vi "tui_DataLog Tag Manager.vi"() -> ()   [LabVIEW 2012]
doc: "Manages tags contained in the logging databases present on the connected server. This manager requires that the \"Databases Module\" is initialised on the server. The operations allowed on the selected database depend on the mode of that database. \n\nIf you find yourself repeatedly performing the same kinds of operations, e.g. because the number of tags in a database is very large, some automation might be handy. For this reason, the management operations can also be performed programatically by calling export functions of the \"Databases Module\" from a script."
uses:
  typedefs/t_Datalog Datebase Modes.ctl
  served/DataLog Database Infos_srv.ctl
  served/DataLog Tag Subset Last_srv.ctl
  served/DataLog Databases_srv.ctl
  served/DataLog Set Tag Value_srv.ctl
  served/DataLog Dump Tag Buffer_srv.ctl
  typedefs/t_DataLog Tag Manager States.ctl
  typedefs/et_DataLog Meta Tag Specifier.ctl
  library/typedefs/t_Library Session Methods.ctl
  typedefs/t_DataLog Tag Info List Methods.ctl
  clientsrv/typedefs/t_ClientSrv Access Levels.ctl
  typedefs/t_DataLog Value Types.ctl
  typedefs/t_DataLog Temporal Types.ctl
panel:
  out "dump tag buffer":T1
  in  "stats":bool
  out "set tag value":T2
  out "mode":T3
  in  "database":i32(ring)
  out "databases":T4
  out "tag subset last":T5
  out "database infos":T6
  in  "set":bool
  in  "chart":bool
  out "total tags":i32
  out "shown tags":i32
  in  "filter/subset":string(combo)
  in  "hide meta?":bool
  in  "selected":string
  in  "configure":bool
  in  "delete":bool
  in  "rename":bool
  in  "clone":bool
  in  "create meta":bool
  in  "create":bool
  in  "tag list":i32(listbox)
  in  "exit":bool
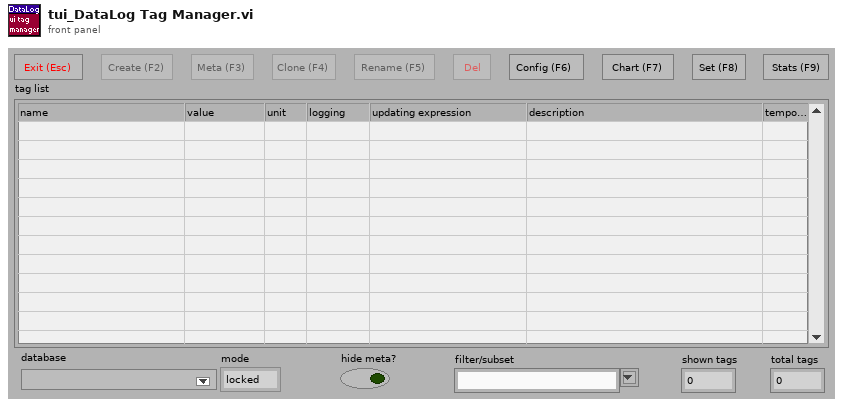
[diagram p1: front panel]
types:
  T1 = typedef "DataLog Dump Tag Buffer_srv.ctl" = refnum<vi>
  T2 = typedef "DataLog Set Tag Value_srv.ctl" = refnum<vi>
  T3 = typedef "t_Datalog Datebase Modes.ctl" = enum16{"locked", "unlocked", "live", "mirrored"}
  T4 = typedef "DataLog Databases_srv.ctl" = refnum<vi>
  T5 = typedef "DataLog Tag Subset Last_srv.ctl" = refnum<vi>
  T6 = typedef "DataLog Database Infos_srv.ctl" = refnum<vi>
  T7 = typedef "et_DataLog Meta Tag Specifier.ctl" = enum32{"warn_lo", "warn_hi", "A_lo", "A_hi", "B_lo", "B_hi", "C_lo", "C_hi", "D_lo", "D_hi", "E_lo", "E_hi", "F_lo", "F_hi", "G_lo", "G_hi", "H_lo", "H_hi", "I_lo", "I_hi", "J_lo", "J_hi", "K_lo", "K_hi", "L_lo", "L_hi", "M_lo", "M_hi", "N_lo", "N_hi", "min", "max", "not a meta"}
  T8 = typedef "t_DataLog Tag Manager States.ctl" = enum16{"empty queue", "poll list", "poll live", "resize", "set database", "get subsets", "winnow list", "filter list", "subset list", "show list", "create tag", "create meta tag", "clone tag", "rename tag", "configure tag", "chart tag", "set tag", "stat tag", "delete tag", "ablement", "initialize", "init refs", "init databases", "init persist", "cleanup", "stop"}
  T9 = typedef "t_Library Session Methods.ctl" = enum16{"run", "get arg", "set arg", "delist", "cleanup?", "start session", "stop session", "list empty?"}
  T10 = typedef "t_DataLog Tag Info List Methods.ctl" = enum16{"initialize", "create", "create empty", "rename", "delete", "test tag", "get", "get by name", "get default", "get list", "get path", "get subsets", "set subsets", "set config", "set capacity", "#tags", "go live", "set unlocked", "set mirrored"}
  T11 = typedef "t_ClientSrv Access Levels.ctl" = enum16{"observer", "operator", "local"}
  T12 = typedef "t_DataLog Temporal Types.ctl" = enum16{"set&hold", "sample", "event"}
  T13 = typedef "t_DataLog Value Types.ctl" = enum16{"number", "string"}
  T14 = typedef "eventvkey.ctl" = enum16{"ASCII", "Enter", "Return", "Shift", "Ctrl", "Alt", "Cmd", "Opt", "Caps", "NumLock", "Clear", "Break", "Up", "Down", "Left", "Right", "Insert", "Delete", "Home", "End", "PageUp", "PageDown", "Escape", "Help", "Pause", "ScrollLock", "F1", "F2", "F3", "F4", "F5", "F6", "F7", "F8", "F9", "F10", "F11", "F12", "F13", "F14", "F15", "F16", "F17", "F18", "F19", "F20", "F21", "F22", "F23", "F24", "Play", "VolumeUp", "VolumeDown", "Mute", "Two Byte Char"}
  T15 = typedef "t_DataLog Tag Config.ctl" = cluster{"name":string, "unit":string, "temporal":T12, "value":T13, "index":i32, "capacity":i32, "is meta?":bool, "mincapacity":i32, "deadband":dbl, "limit delay":dbl, "format":T16, "precision":u8, "undefine":bool, "update":bool, "update period":u16, "expression":string, "description":string, "logging algorithm":T17, "logging parameters":dbl[]}
  T16 = typedef "t_DataLog Numerical Format.ctl" = enum8{"fractional", "exponential", "engineering"}
  T17 = typedef "t_DataLog Logging Algorithms.ctl" = enum16{"nothing", "changes", "everything", "every Nth", "time threshold", "value threshold + prior", "t or v threshold", "t or v threshold + prior"}
  T18 = typedef "LVRowAndColumnUnsignedTypeDef.ctl" = cluster{"Row":u32, "Column":u32}
  T19 = typedef "t_DataLog Tag Subset.ctl" = cluster{"name":string, "tags":string[]}
  T20 = typedef "t_DataLog Point.ctl" = cluster{"time":dbl, "value":dbl}
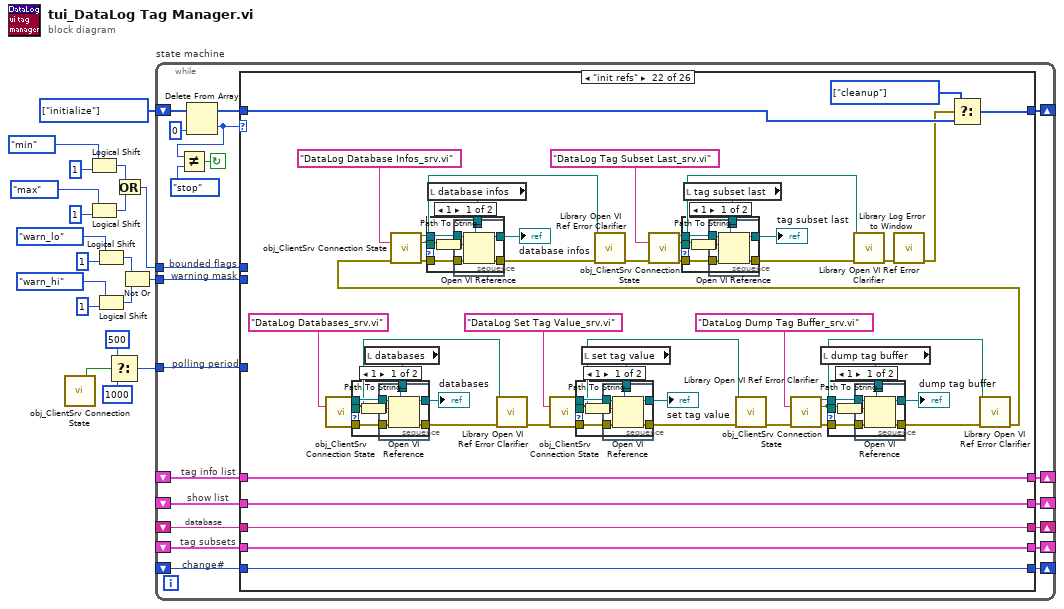
[diagram p0: block diagram]
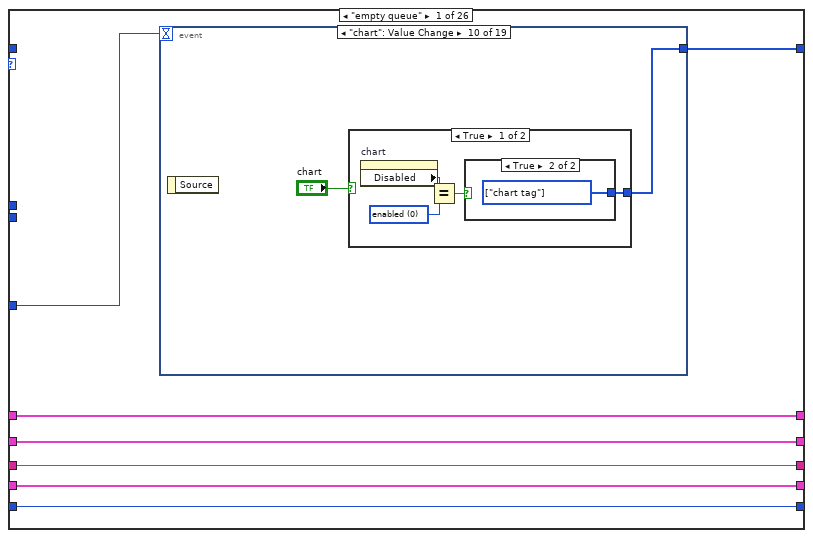
[diagram p2: hidden frame]
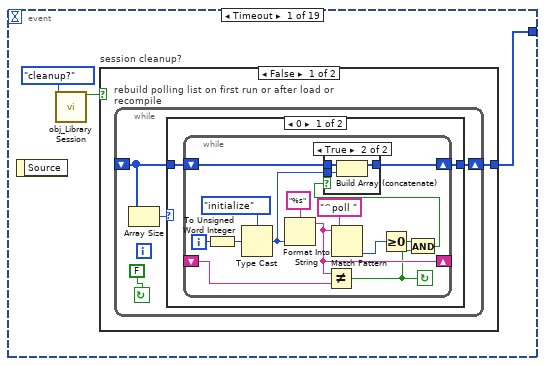
[diagram p3: hidden frame]
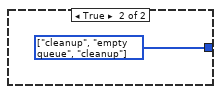
[diagram p6: hidden frame]
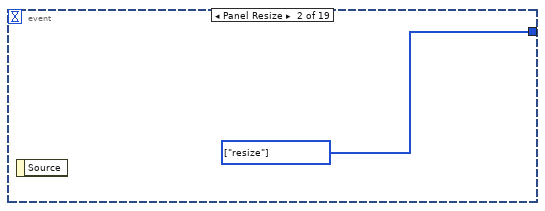
[diagram p7: hidden frame]
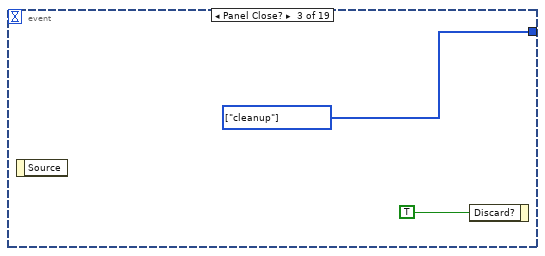
[diagram p8: hidden frame]
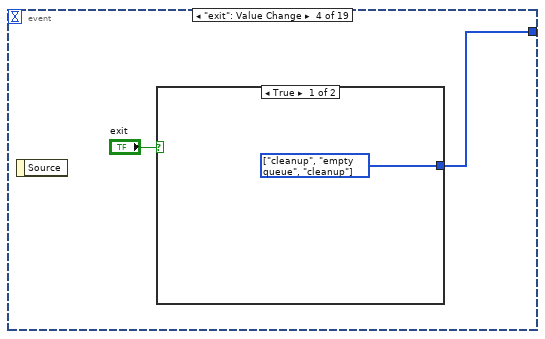
[diagram p9: hidden frame]
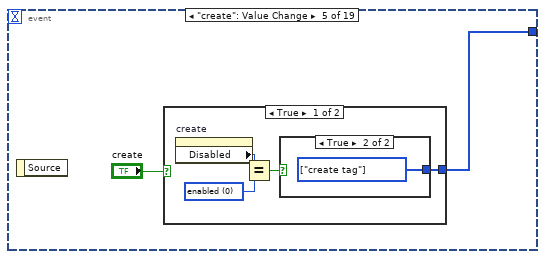
[diagram p11: hidden frame]
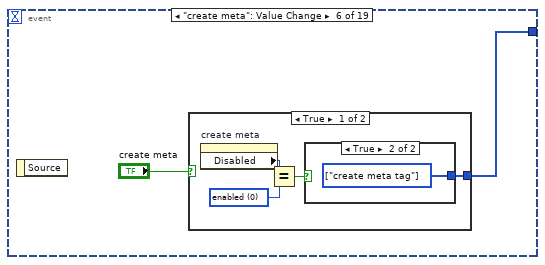
[diagram p14: hidden frame]
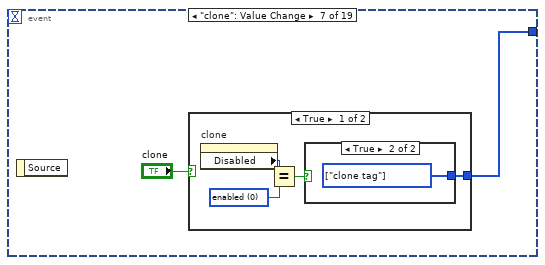
[diagram p17: hidden frame]
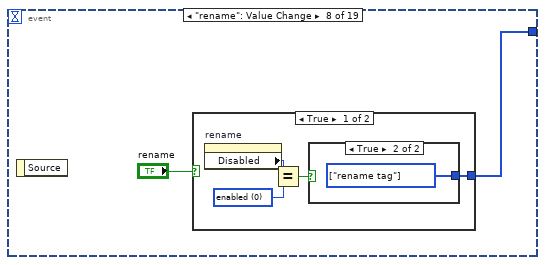
[diagram p20: hidden frame]
diagram:
  w19 = T8[] [enum."initialize"] items=["empty queue", "poll list", "poll live", "resize", "set database", "get subsets", "winnow list", "filter list", "subset list", "show list", "create tag", "create meta tag", "clone tag", "rename tag", "configure tag", "chart tag", "set tag", "stat tag", "delete tag", "ablement", "initialize", "init refs", "init databases", "init persist", "cleanup", "stop"] ("Array Constant")
  n1 = call "obj_ClientSrv Connection State.vi"() -> ("local?"=w9:bool)  [unwired: 8 in, 7 out]
  n2 = Logical Shift(y=et_DataLog_Meta_Tag_Specifier."min" ("meta specifier"), x=u32 1) -> (x << y=w6:u32)
  n3 = Logical Shift(y=et_DataLog_Meta_Tag_Specifier."max" ("meta specifier"), x=u32 1) -> (x << y=w7:u32)
  n4 = Logical Shift(y=et_DataLog_Meta_Tag_Specifier."warn_lo" ("meta specifier"), x=u32 1) -> (x << y=w14:u32)
  n5 = Logical Shift(y=et_DataLog_Meta_Tag_Specifier."warn_hi" ("meta specifier"), x=u32 1) -> (x << y=w13:u32)
  n6 = Select(t=500, s=w9, f=1000) -> (s? t:f=w8:i32)
  n7 = Or(x=w6, y=w7) -> (x .or. y?=w1:u32)
  n8 = Not Or(1:w13, 2:w14) -> (0:w12:u32)
  n9 = while "state machine" {
    shift-left: w19 -> [w36]
    shift-right: [w39] -> _
    shift-right: [w32] -> _
    shift-left: _ -> [w33]
    shift-right: [w30] -> _
    shift-left: _ -> [w31]
    tunnel: w12 -> [w29]
    tunnel: w8 -> [w27]
    shift-right: [w25] -> _
    shift-left: _ -> [w26]
    tunnel: w1 -> [w24]
    shift-right: [w23] -> _
    shift-left: _ -> [w22]
    shift-right: [w20] -> _
    shift-left: _ -> [w21]
    stop <- w38 continue-if-true
    # "change#"
    # "tag subsets"
    # "bounded flags"
    # "database"
    # "polling period"
    # "warning mask"
    # "show list"
    # "tag info list"
    n10 = Delete From Array(array=w36, index=0) -> (deleted portion=w28:T8, array with subset deleted=w35:T8[])  [unwired: 1 in]
    n11 = Not Equal?(x=w28, y=t_DataLog_Tag_Manager_States."stop" ("states")) -> (x != y?=w38:bool)
    n12 = case "Case" shown="\"init refs\"" w28 {
      tunnel: [w46 w178 w231 w303 w310 w335 w375 w391 w426 w474 w535 w599 w642 w672 w694 w734 w747 w774 w795 w844 w859 w937 w1052 w1062 w1092 w1098] -> w39
      tunnel: w35 -> [_ w179 w231 w303 w310 w334 w374 w390 w425 w473 w534 w598 w641 w671 _ w734 w745 w774 w794 w844 _ w935 w1043 w1063 _ w1098]
      tunnel: w33 -> [w45 w180 w229 w305 w315 w347 w371 _ _ w470 w539 w601 w638 w674 w697 w737 w750 w778 w797 w840 w863 w934 w1060 w1069 w1083 w1097]
      tunnel: [w45 w180 w228 w305 w315 w347 w371 w383 w421 w470 w539 w601 w638 w674 w697 w737 w750 w778 w797 w840 w863 w934 w1060 w1069 w1082 w1097] -> w32
      tunnel: w31 -> [w44 w182 w232 w304 w314 w346 w370 w385 w422 w471 w533 w595 w640 w664 w695 w735 w748 w776 w787 w842 w862 w933 w1059 w1068 w1091 w1096]
      tunnel: [w44 w181 w232 w304 w314 w346 w370 w386 w423 w471 w533 w595 w640 w664 w695 w735 w748 w776 w787 w842 w862 w933 w1059 w1068 w1086 w1096] -> w30
      tunnel: w29 -> [_ _ w227 _ _ _ _ _ _ _ _ _ _ _ _ _ _ _ _ _ _ _ _ _ _ _]
      tunnel: w27 -> [w43 _ _ _ _ _ _ _ _ _ _ _ _ _ _ _ _ _ _ _ _ _ _ _ _ _]
      tunnel: w26 -> [w42 w168 w226 w301 _ w328 w373 w379 w420 w469 w532 w594 w635 w663 w692 w727 w744 w775 w786 w818 w861 w926 w1046 w1067 w1080 w1095]
      tunnel: [w42 w168 w226 w301 w306 w328 w373 w379 w420 w469 w532 w594 w635 w663 w692 w727 w744 w775 w786 w818 w861 w926 w1046 w1067 w1080 w1095] -> w25
      tunnel: w24 -> [_ _ w225 _ _ _ _ _ _ _ _ _ _ _ _ _ _ _ _ _ _ _ _ _ _ _]
      tunnel: [w41 w167 w224 w300 w312 w339 w372 w378 w416 w468 w531 w592 w634 w662 w691 w726 w739 w764 w784 w812 w860 w920 w1047 w1066 w1071 w1094] -> w23
      tunnel: w22 -> [w41 w167 w224 w300 w312 _ w372 w378 w416 w468 w531 w592 w634 w662 w691 w726 w739 w764 w784 w812 w860 w920 w1047 w1066 w1071 w1094]
      tunnel: w21 -> [w40 w166 w223 w299 _ w329 w363 w376 w412 w467 w530 w591 w633 w661 w690 w725 w738 w763 w783 w811 w858 w919 w1045 w1064 w1070 w1093]
      tunnel: [w40 w165 w223 w299 0 ("#tags") w329 w363 w376 w412 w467 w530 w591 w633 w661 w690 w725 w738 w763 w783 w811 w858 w919 w1045 w1064 w1070 w1093] -> w20
      frame "empty queue" {
        n13 = event shown="[9] \"chart\": Value Change" {
          selector: _ -> [_ _ _ _ _ _ _ _ _ _ _ _ _ _ _ _ _ _ _]
          dyn-events: _ -> [_ _ _ _ _ _ _ _ _ _ _ _ _ _ _ _ _ _ _]
          timeout: w43 -> [_ _ _ _ _ _ _ _ _ _ _ _ _ _ _ _ _ _ _]
          tunnel: [w49 w77 w79 w81 w83 w90 w97 w104 w111 w119 w126 w133 w139 w146 w147 w148 w149 _ _] -> w46
          event Timeout {
            n14 = event-data() -> ()  [unwired: 1 in, 1 out]
            n15 = call "obj_Library Session.vi"("method"=t_Library_Session_Methods."cleanup?") -> ("cleanup/empty?"=w47:bool)  [unwired: 11 in, 3 out]
            n16 = case "session cleanup?" shown="False" w47 {
              tunnel: [w50 w76] -> w49
              frame False {
                n17 = while "rebuild polling list on first run or after load or recompile" {
                  shift-left: _ -> [w53]
                  shift-right: [w52] -> w50
                  stop <- FALSE continue-if-true
                  n18 = Array Size(array=w53) -> (size(s)=w54:i32)
                  n19 = case shown="0" w54 {
                    tunnel: [w55 w75] -> w52
                    tunnel: w53 -> [w56 w75]
                    frame 0 {
                      n20 = while {
                        shift-left: w56 -> [w65]
                        shift-right: [w63] -> w55
                        shift-left: _ -> [w67]
                        shift-right: [w62] -> _
                        i -> [w70]
                        stop <- w58 continue-if-true
                        n21 = To Unsigned Word Integer(number=w70) -> (unsigned 16bit integer=w68:u16)
                        n22 = Type Cast(type=t_DataLog_Tag_Manager_States."initialize" ("states"), x=w68) -> (*(type *) &x=w64:T8)
                        n23 = Format Into String(format string="%s" ("Format String"), w64) -> (resulting string=w62:string)  [unwired: 2 in, 1 out]
                        n24 = Not Equal?(x=w62, y=w67) -> (x != y?=w58:bool)
                        n25 = Match Pattern(string=w62, regular expression="^poll ") -> (offset past match=w60:i32)  [unwired: 1 in, 3 out]
                        n26 = Greater Or Equal To 0?(x=w60) -> (x >= 0?=w59:bool)
                        n27 = And(x=w59, y=w58) -> (x .and. y?=w57:bool)
                        n28 = case shown="True" w57 {
                          tunnel: w65 -> [w71 w74]
                          tunnel: w64 -> [_ w73]
                          tunnel: [w71 w72] -> w63
                          frame False {
                          }
                          frame True {
                            n29 = Build Array (concatenate)(w74, w73) -> (w72:T8[])
                          }
                        }
                      }
                    }
                    frame Default {
                    }
                  }
                }
              }
              frame True {
                w76 = T8[] [enum."cleanup", enum."empty queue", enum."cleanup"] items=["empty queue", "poll list", "poll live", "resize", "set database", "get subsets", "winnow list", "filter list", "subset list", "show list", "create tag", "create meta tag", "clone tag", "rename tag", "configure tag", "chart tag", "set tag", "stat tag", "delete tag", "ablement", "initialize", "init refs", "init databases", "init persist", "cleanup", "stop"] ("Array Constant")
              }
            }
          }
          event Panel Resize {
            w77 = T8[] [enum."resize"] items=["empty queue", "poll list", "poll live", "resize", "set database", "get subsets", "winnow list", "filter list", "subset list", "show list", "create tag", "create meta tag", "clone tag", "rename tag", "configure tag", "chart tag", "set tag", "stat tag", "delete tag", "ablement", "initialize", "init refs", "init databases", "init persist", "cleanup", "stop"] ("Array Constant")
            n30 = event-data() -> ()  [unwired: 1 in, 1 out]
          }
          event Panel Close? {
            w79 = T8[] [enum."cleanup"] items=["empty queue", "poll list", "poll live", "resize", "set database", "get subsets", "winnow list", "filter list", "subset list", "show list", "create tag", "create meta tag", "clone tag", "rename tag", "configure tag", "chart tag", "set tag", "stat tag", "delete tag", "ablement", "initialize", "init refs", "init databases", "init persist", "cleanup", "stop"] ("Array Constant")
            n31 = event-data() -> ()  [unwired: 1 in, 1 out]
            n32 = event-data("Discard?"=TRUE) -> ()  [unwired: 1 in, 1 out]
          }
          event "exit": Value Change {
            n33 = event-data() -> ()  [unwired: 1 in, 1 out]
            n34 = case shown="True" "exit" {
              tunnel: [w82 _] -> w81
              frame True {
                w82 = T8[] [enum."cleanup", enum."empty queue", enum."cleanup"] items=["empty queue", "poll list", "poll live", "resize", "set database", "get subsets", "winnow list", "filter list", "subset list", "show list", "create tag", "create meta tag", "clone tag", "rename tag", "configure tag", "chart tag", "set tag", "stat tag", "delete tag", "ablement", "initialize", "init refs", "init databases", "init persist", "cleanup", "stop"] ("Array Constant")
              }
              frame False {
              }
            }
          }
          event "create": Value Change {
            n35 = event-data() -> ()  [unwired: 1 in, 1 out]
            n36 = case shown="True" "create" {
              tunnel: [w88 _] -> w83
              frame True {
                w87 = u8 0 items=["enabled", "disabled", "grayed"] ("disabled state")
                n37 = property on="create" class="Bool"() -> ("Disabled"=w86:u8)  [unwired: 2 in, 2 out]
                n38 = Equal?(x=w86, y=w87) -> (x = y?=w85:bool)
                n39 = case shown="True" w85 {
                  tunnel: [_ w89] -> w88
                  frame False {
                  }
                  frame True {
                    w89 = T8[] [enum."create tag"] items=["empty queue", "poll list", "poll live", "resize", "set database", "get subsets", "winnow list", "filter list", "subset list", "show list", "create tag", "create meta tag", "clone tag", "rename tag", "configure tag", "chart tag", "set tag", "stat tag", "delete tag", "ablement", "initialize", "init refs", "init databases", "init persist", "cleanup", "stop"] ("Array Constant")
                  }
                }
              }
              frame False {
              }
            }
          }
          event "create meta": Value Change {
            n40 = event-data() -> ()  [unwired: 1 in, 1 out]
            n41 = case shown="True" "create meta" {
              tunnel: [w95 _] -> w90
              frame True {
                w94 = u8 0 items=["enabled", "disabled", "grayed"] ("disabled state")
                n42 = property on="create meta" class="Bool"() -> ("Disabled"=w93:u8)  [unwired: 2 in, 2 out]
                n43 = Equal?(x=w93, y=w94) -> (x = y?=w92:bool)
                n44 = case shown="True" w92 {
                  tunnel: [_ w96] -> w95
                  frame False {
                  }
                  frame True {
                    w96 = T8[] [enum."create meta tag"] items=["empty queue", "poll list", "poll live", "resize", "set database", "get subsets", "winnow list", "filter list", "subset list", "show list", "create tag", "create meta tag", "clone tag", "rename tag", "configure tag", "chart tag", "set tag", "stat tag", "delete tag", "ablement", "initialize", "init refs", "init databases", "init persist", "cleanup", "stop"] ("Array Constant")
                  }
                }
              }
              frame False {
              }
            }
          }
          event "clone": Value Change {
            n45 = event-data() -> ()  [unwired: 1 in, 1 out]
            n46 = case shown="True" "clone" {
              tunnel: [w102 _] -> w97
              frame True {
                w101 = u8 0 items=["enabled", "disabled", "grayed"] ("disabled state")
                n47 = property on="clone" class="Bool"() -> ("Disabled"=w100:u8)  [unwired: 2 in, 2 out]
                n48 = Equal?(x=w100, y=w101) -> (x = y?=w99:bool)
                n49 = case shown="True" w99 {
                  tunnel: [_ w103] -> w102
                  frame False {
                  }
                  frame True {
                    w103 = T8[] [enum."clone tag"] items=["empty queue", "poll list", "poll live", "resize", "set database", "get subsets", "winnow list", "filter list", "subset list", "show list", "create tag", "create meta tag", "clone tag", "rename tag", "configure tag", "chart tag", "set tag", "stat tag", "delete tag", "ablement", "initialize", "init refs", "init databases", "init persist", "cleanup", "stop"] ("Array Constant")
                  }
                }
              }
              frame False {
              }
            }
          }
          event "rename": Value Change {
            n50 = event-data() -> ()  [unwired: 1 in, 1 out]
            n51 = case shown="True" "rename" {
              tunnel: [w109 _] -> w104
              frame True {
                w108 = u8 0 items=["enabled", "disabled", "grayed"] ("disabled state")
                n52 = property on="rename" class="Bool"() -> ("Disabled"=w107:u8)  [unwired: 2 in, 2 out]
                n53 = Equal?(x=w107, y=w108) -> (x = y?=w106:bool)
                n54 = case shown="True" w106 {
                  tunnel: [_ w110] -> w109
                  frame False {
                  }
                  frame True {
                    w110 = T8[] [enum."rename tag"] items=["empty queue", "poll list", "poll live", "resize", "set database", "get subsets", "winnow list", "filter list", "subset list", "show list", "create tag", "create meta tag", "clone tag", "rename tag", "configure tag", "chart tag", "set tag", "stat tag", "delete tag", "ablement", "initialize", "init refs", "init databases", "init persist", "cleanup", "stop"] ("Array Constant")
                  }
                }
              }
              frame False {
              }
            }
          }
          event "configure": Value Change {
            n55 = event-data() -> ()  [unwired: 1 in, 1 out]
            n56 = case shown="True" "configure" {
              tunnel: [w116 _] -> w111
              frame True {
                w115 = u8 0 items=["enabled", "disabled", "grayed"] ("disabled state")
                n57 = property on="configure" class="Bool"() -> ("Disabled"=w114:u8)  [unwired: 2 in, 2 out]
                n58 = Equal?(x=w114, y=w115) -> (x = y?=w113:bool)
                n59 = case shown="True" w113 {
                  tunnel: [_ w117] -> w116
                  frame False {
                  }
                  frame True {
                    w117 = T8[] [enum."configure tag"] items=["empty queue", "poll list", "poll live", "resize", "set database", "get subsets", "winnow list", "filter list", "subset list", "show list", "create tag", "create meta tag", "clone tag", "rename tag", "configure tag", "chart tag", "set tag", "stat tag", "delete tag", "ablement", "initialize", "init refs", "init databases", "init persist", "cleanup", "stop"] ("Array Constant")
                  }
                }
              }
              frame False {
              }
            }
          }
          event "chart": Value Change {
            n60 = event-data() -> ()  [unwired: 1 in, 1 out]
            n61 = case shown="True" "chart" {
              tunnel: [w123 _] -> w119
              frame True {
                w122 = u8 0 items=["enabled", "disabled", "grayed"] ("disabled state")
                n62 = property on="chart" class="Bool"() -> ("Disabled"=w121:u8)  [unwired: 2 in, 2 out]
                n63 = Equal?(x=w121, y=w122) -> (x = y?=w120:bool)
                n64 = case shown="True" w120 {
                  tunnel: [_ w124] -> w123
                  frame False {
                  }
                  frame True {
                    w124 = T8[] [enum."chart tag"] items=["empty queue", "poll list", "poll live", "resize", "set database", "get subsets", "winnow list", "filter list", "subset list", "show list", "create tag", "create meta tag", "clone tag", "rename tag", "configure tag", "chart tag", "set tag", "stat tag", "delete tag", "ablement", "initialize", "init refs", "init databases", "init persist", "cleanup", "stop"] ("Array Constant")
                  }
                }
              }
              frame False {
              }
            }
          }
          event "set": Value Change {
            n65 = event-data() -> ()  [unwired: 1 in, 1 out]
            n66 = case shown="True" "set" {
              tunnel: [w130 _] -> w126
              frame True {
                w129 = u8 0 items=["enabled", "disabled", "grayed"] ("disabled state")
                n67 = property on="set" class="Bool"() -> ("Disabled"=w128:u8)  [unwired: 2 in, 2 out]
                n68 = Equal?(x=w128, y=w129) -> (x = y?=w127:bool)
                n69 = case shown="True" w127 {
                  tunnel: [_ w131] -> w130
                  frame False {
                  }
                  frame True {
                    w131 = T8[] [enum."set tag"] items=["empty queue", "poll list", "poll live", "resize", "set database", "get subsets", "winnow list", "filter list", "subset list", "show list", "create tag", "create meta tag", "clone tag", "rename tag", "configure tag", "chart tag", "set tag", "stat tag", "delete tag", "ablement", "initialize", "init refs", "init databases", "init persist", "cleanup", "stop"] ("Array Constant")
                  }
                }
              }
              frame False {
              }
            }
          }
          event "stats": Value Change {
            n70 = event-data() -> ()  [unwired: 1 in, 1 out]
            n71 = case shown="True" "stats" {
              tunnel: [w137 _] -> w133
              frame True {
                w136 = u8 0 items=["enabled", "disabled", "grayed"] ("disabled state")
                n72 = property on="stats" class="Bool"() -> ("Disabled"=w135:u8)  [unwired: 2 in, 2 out]
                n73 = Equal?(x=w135, y=w136) -> (x = y?=w134:bool)
                n74 = case shown="True" w134 {
                  tunnel: [_ w138] -> w137
                  frame False {
                  }
                  frame True {
                    w138 = T8[] [enum."stat tag"] items=["empty queue", "poll list", "poll live", "resize", "set database", "get subsets", "winnow list", "filter list", "subset list", "show list", "create tag", "create meta tag", "clone tag", "rename tag", "configure tag", "chart tag", "set tag", "stat tag", "delete tag", "ablement", "initialize", "init refs", "init databases", "init persist", "cleanup", "stop"] ("Array Constant")
                  }
                }
              }
              frame False {
              }
            }
          }
          event "delete": Value Change {
            n75 = event-data() -> ()  [unwired: 1 in, 1 out]
            n76 = case shown="True" "delete" {
              tunnel: [w144 _] -> w139
              frame True {
                w143 = u8 0 items=["enabled", "disabled", "grayed"] ("disabled state")
                n77 = property on="delete" class="Bool"() -> ("Disabled"=w142:u8)  [unwired: 2 in, 2 out]
                n78 = Equal?(x=w142, y=w143) -> (x = y?=w141:bool)
                n79 = case shown="True" w141 {
                  tunnel: [_ w145] -> w144
                  frame False {
                  }
                  frame True {
                    w145 = T8[] [enum."delete tag"] items=["empty queue", "poll list", "poll live", "resize", "set database", "get subsets", "winnow list", "filter list", "subset list", "show list", "create tag", "create meta tag", "clone tag", "rename tag", "configure tag", "chart tag", "set tag", "stat tag", "delete tag", "ablement", "initialize", "init refs", "init databases", "init persist", "cleanup", "stop"] ("Array Constant")
                  }
                }
              }
              frame False {
              }
            }
          }
          event "tag list": Value Change {
            w146 = T8[] [enum."ablement"] items=["empty queue", "poll list", "poll live", "resize", "set database", "get subsets", "winnow list", "filter list", "subset list", "show list", "create tag", "create meta tag", "clone tag", "rename tag", "configure tag", "chart tag", "set tag", "stat tag", "delete tag", "ablement", "initialize", "init refs", "init databases", "init persist", "cleanup", "stop"] ("Array Constant")
            n80 = event-data() -> ()  [unwired: 1 in, 1 out]
          }
          event "hide meta?": Value Change {
            w147 = T8[] [enum."winnow list"] items=["empty queue", "poll list", "poll live", "resize", "set database", "get subsets", "winnow list", "filter list", "subset list", "show list", "create tag", "create meta tag", "clone tag", "rename tag", "configure tag", "chart tag", "set tag", "stat tag", "delete tag", "ablement", "initialize", "init refs", "init databases", "init persist", "cleanup", "stop"] ("Array Constant")
            n81 = event-data() -> ()  [unwired: 1 in, 1 out]
          }
          event "filter/subset": Value Change {
            w148 = T8[] [enum."winnow list"] items=["empty queue", "poll list", "poll live", "resize", "set database", "get subsets", "winnow list", "filter list", "subset list", "show list", "create tag", "create meta tag", "clone tag", "rename tag", "configure tag", "chart tag", "set tag", "stat tag", "delete tag", "ablement", "initialize", "init refs", "init databases", "init persist", "cleanup", "stop"] ("Array Constant")
            n82 = event-data() -> ()  [unwired: 1 in, 1 out]
          }
          event "database": Value Change {
            w149 = T8[] [enum."set database", enum."get subsets", enum."poll list"] items=["empty queue", "poll list", "poll live", "resize", "set database", "get subsets", "winnow list", "filter list", "subset list", "show list", "create tag", "create meta tag", "clone tag", "rename tag", "configure tag", "chart tag", "set tag", "stat tag", "delete tag", "ablement", "initialize", "init refs", "init databases", "init persist", "cleanup", "stop"] ("Array Constant")
            n83 = event-data() -> ()  [unwired: 1 in, 1 out]
          }
          event Key Down? {
            n84 = event-data() -> ("VKey"=w150:T14, "FocusObj"=w151:refnum<vi>)  [unwired: 1 in]
            n85 = call <vilib>:"compatReturnToEnter.vi"("VKey"=w150) -> ("VKey"=w153:T14)
            n86 = case shown="\"Up\", \"Down\"" w153 {
              tunnel: [_ TRUE _] -> w152
              tunnel: w151 -> [w157 _ _]
              frame "Up", "Down" {
                n87 = Type Cast(type=u32 0, x=w157) -> (*(type *) &x=w155:u32)
                n88 = Equal To 0?(x=w155) -> (x = 0?=w154:bool)
                n89 = case shown="True" w154 {
                  frame False {
                  }
                  frame True {
                    n90 = property on="tag list" class="MCListbox (strict)"("Key Focus"=TRUE) -> ()  [unwired: 2 in, 2 out]
                  }
                }
              }
              frame "F1" {
                n91 = call "Library Show Help.vi"() -> ()  [unwired: 1 in]
              }
              frame Default {
              }
            }
            n92 = event-data("Discard?"=w152) -> ()  [unwired: 1 in, 1 out]
          }
          event event type 5.0.x8000000b {
            n93 = event-data() -> ("VKey"=w160:T14)  [unwired: 1 in]
            n94 = call <vilib>:"compatReturnToEnter.vi"("VKey"=w160) -> ("VKey"=w162:T14)
            n95 = case shown="\"F1\"" w162 {
              tunnel: [TRUE _] -> w161
              frame "F1" {
              }
              frame Default {
              }
            }
            n96 = event-data("Discard?"=w161) -> ()  [unwired: 1 in, 1 out]
          }
        }
      }
      frame "poll list" {
        n97 = local read "database infos"() -> (w172:T6)
        n98 = call "obj_ClientSrv Client Access State.vi"() -> ("certificate"=w170:string, "error out"=w173:errorcluster)  [unwired: 14 in]
        n99 = call-by-ref "?"(reference=w172, error in=w173, "method"=t_DataLog_Tag_Info_List_Methods."get list", "meta specifier (not a meta)"=w166, "certificate in"=w170, "database (current)"=w168) -> (error out=w174:errorcluster, "mode"=w176:T3, "tag config list"=w175:T15[], "#tags/change#"=w164:i32, 15:"error out"=w171:errorcluster)  [unwired: 6 in, 3 out]
        n100 = call "Library Remote Call Error Merger.vi"("call by reference node error"=w174, "called VI error (no error)"=w171) -> ("error out"=w169:errorcluster)  [unwired: 13 in]
        n101 = case shown="No Error" w169 {
          selector: w169 -> [_ w220]
          tunnel: w182 -> [w192 w221]
          tunnel: [w191 w221] -> w181
          tunnel: w179 -> [w190 _]
          tunnel: [w189 w222] -> w178
          tunnel: w176 -> [w188 _]
          tunnel: w175 -> [w187 _]
          tunnel: w166 -> [w185 w219]
          tunnel: [w184 w219] -> w165
          tunnel: w164 -> [w183 _]
          frame No Error {
            n102 = Not Equal?(x=w183, y=w185) -> (x != y?=w194:bool)
            n103 = Equal To 0?(x=w185) -> (x = 0?=w186:bool)
            n104 = Or(x=w194, y=w186) -> (x .or. y?=w193:bool)
            n105 = case shown="False" w193 {
              tunnel: [w201 w215] -> w191
              tunnel: w187 -> [_ w215]
              tunnel: w192 -> [w201 _]
              tunnel: w190 -> [w198 w217]
              tunnel: w188 -> [w200 w218]
              tunnel: [w197 w216] -> w189
              tunnel: w185 -> [w195 _]
              tunnel: [w195 w213] -> w184
              tunnel: w183 -> [_ w213]
              frame False {
                n106 = local read "mode"() -> (w196:T3)
                n107 = Not Equal?(x=w200, y=w196) -> (x != y?=w199:bool)
                n108 = case shown="True" w199 {
                  tunnel: w200 -> [_ w203]
                  tunnel: w198 -> [w202 w205]
                  tunnel: [w202 w204] -> w197
                  frame False {
                  }
                  frame True {
                    n109 = case shown="\"locked\", \"unlocked\", \"mirrored\"" w203 {
                      tunnel: w205 -> [w207 w210]
                      tunnel: [w206 w209] -> w204
                      frame "locked", "unlocked", "mirrored" {
                        n110 = Build Array (concatenate)(t_DataLog_Tag_Manager_States."show list" ("states"), w207) -> (w206:T8[])
                      }
                      frame "live" {
                        n111 = Build Array (concatenate)(t_DataLog_Tag_Manager_States."ablement" ("states"), w210) -> (w209:T8[])
                      }
                    }
                    "mode" <- w203
                  }
                }
              }
              frame True {
                w212 = T8[] [enum."get subsets", enum."winnow list"] items=["empty queue", "poll list", "poll live", "resize", "set database", "get subsets", "winnow list", "filter list", "subset list", "show list", "create tag", "create meta tag", "clone tag", "rename tag", "configure tag", "chart tag", "set tag", "stat tag", "delete tag", "ablement", "initialize", "init refs", "init databases", "init persist", "cleanup", "stop"] ("Array Constant")
                # "might be the subsets that have changed"
                n112 = local write "mode"(w218) -> ()
                n113 = Array Size(array=w215) -> (size(s)=→"total tags":i32)
                n114 = Build Array (concatenate)(w212, w217) -> (w216:T8[])
              }
            }
          }
          frame Error {
            w222 = T8[] [enum."cleanup"] items=["empty queue", "poll list", "poll live", "resize", "set database", "get subsets", "winnow list", "filter list", "subset list", "show list", "create tag", "create meta tag", "clone tag", "rename tag", "configure tag", "chart tag", "set tag", "stat tag", "delete tag", "ablement", "initialize", "init refs", "init databases", "init persist", "cleanup", "stop"] ("Array Constant")
            n115 = call "Library Log Error to Window.vi"("error in (no error)"=w220) -> ()  [unwired: 13 in, 2 out]
          }
        }
      }
      frame "poll live" {
        n116 = local read "mode"() -> (w230:T3)
        n117 = case shown="\"live\"" w230 {
          tunnel: w229 -> [w233 w237]
          tunnel: [w233 w234] -> w228
          tunnel: w227 -> [_ w236]
          tunnel: w225 -> [_ w235]
          frame Default {
          }
          frame "live" {
            n118 = stacked-sequence {
              tunnel: w237 -> [_ w248 _]
              tunnel: w236 -> [_ w257 _]
              tunnel: w235 -> [_ w242 _]
              tunnel: [_ w240 _] -> w234
              frame #0 {
                n119 = property class="VI"() -> ("Front Panel"=w238:refnum<vi>)  [unwired: 2 in, 2 out]
                n120 = property class="Pnl"(reference=w238, "Defer Panel Updates"=TRUE) -> ()  [unwired: 1 in, 2 out]
              }
              frame #1 {
                # "ignore error since\ndatabase might\nbe switching\nmodes."
                n121 = property on="tag list" class="MCListbox (strict)"() -> ("Item Names"=w262:string[][], "Top Left Visible Cell"=w258:T18, "Number of Rows"=w259:u32)  [unwired: 2 in, 2 out]
                n122 = local read "tag subset last"() -> (w255:T5)
                n123 = To Long Integer(number=w259) -> (32bit integer=w244:i32)
                n124 = Unbundle(w258) -> ("Row"=w260:u32)  [unwired: 1 out]
                n125 = Array Size(array=w248) -> (size(s)=w246:i32)
                n126 = To Long Integer(number=w260) -> (32bit integer=w247:i32)
                n127 = Subtract(x=w246, y=w247) -> (x-y=w243:i32)
                n128 = Max & Min(x=w244, y=w243) -> (min(x,y)=w245:i32)  [unwired: 1 out]
                n129 = call "obj_ClientSrv Client Access State.vi"() -> ("certificate"=w254:string, "error out"=w252:errorcluster)  [unwired: 14 in]
                n130 = for {
                  N: w245 -> [_]
                  shift-right: [w294] -> w241
                  shift-left: w248 -> [w294]
                  tunnel: [w293] -> w253 mode=indexing
                  tunnel: [w292] -> w263 mode=indexing
                  tunnel: w247 -> [w291]
                  i -> [w296]
                  n131 = Add(x=w291, y=w296) -> (x+y=w292:i32)
                  n132 = Index Array(array=w294, index=w292) -> (element=w295:T15)
                  n133 = Unbundle By Name(w295) -> ("index"=w293:i32)
                }
                n134 = call-by-ref "?"(reference=w255, error in=w252, "subset indices"=w253, "certificate"=w254) -> (error out=w251:errorcluster, "values"=w250:dbl[], "meta masks"=w249:u32[])  [unwired: 11 in, 2 out]
                n135 = call "Library Remote Call Error Merger.vi"("call by reference node error"=w251) -> ("error out"=w256:errorcluster)  [unwired: 14 in]
                n136 = call "Library Log Error to Window.vi"("error in (no error)"=w256) -> ()  [unwired: 13 in, 2 out]
                n137 = for {
                  tunnel: w263 -> [w266] mode=indexing
                  tunnel: w250 -> [w265] mode=indexing
                  shift-right: [w277] -> w261
                  shift-left: w262 -> [w274]
                  tunnel: w249 -> [w272] mode=indexing
                  tunnel: w257 -> [w271]
                  tunnel: w242 -> [w268]
                  shift-right: [w267] -> w240
                  shift-left: w241 -> [w267]
                  n138 = case shown="Default" w272 {
                    selector: w272 -> [w280 _]
                    tunnel: w271 -> [w282 _]
                    tunnel: [w281 u32 15790320] -> w270
                    tunnel: w268 -> [w279 _]
                    frame Default {
                      n139 = And(x=w280, y=w279) -> (x .and. y?=w278:u32)
                      n140 = case shown="0" w278 {
                        tunnel: w280 -> [w286 _]
                        tunnel: w282 -> [w285 _]
                        tunnel: [w283 u32 16711935] -> w281
                        frame 0 {
                          n141 = And(x=w286, y=w285) -> (x .and. y?=w284:u32)
                          n142 = case shown="0" w284 {
                            tunnel: [u32 16727100 u32 16744448] -> w283
                            frame Default {
                            }
                            frame 0 {
                            }
                          }
                        }
                        frame Default {
                        }
                      }
                    }
                    frame 0 {
                    }
                  }
                  n143 = Index Array(array=w267, index=w266) -> (element=w264:T15)
                  n144 = Bundle(w266, "x+y"=1) -> (w269:cluster{i32, "x+y":i32})  [unwired: 1 in]
                  n145 = call "DataLog Format Point Value.vi"("value"=w265, "tag config"=w264) -> ("formatted value"=w275:string)  [unwired: 13 in]
                  n146 = property on="tag list" class="MCListbox (strict)"("Active Cell:Active Cell"=w269, "Active Cell:Cell Background Color"=w270) -> ()  [unwired: 2 in, 2 out]
                  n147 = Replace Array Subset(array=w274, new element=w275, index (row)=w266, index (col)=1 ("disabled index (col)")) -> (w277:string[][])
                }
                n148 = property on="tag list" class="MCListbox (strict)"("Item Names"=w261) -> ()  [unwired: 2 in, 2 out]
              }
              frame #2 {
                n149 = property class="VI"() -> ("Front Panel"=w297:refnum<vi>)  [unwired: 2 in, 2 out]
                n150 = property class="Pnl"(reference=w297, "Defer Panel Updates"=FALSE) -> ()  [unwired: 1 in, 2 out]
              }
            }
          }
        }
      }
      frame "resize" {
        n151 = control-ref of="tag list"() -> (w302:refnum<vi>)
        n152 = call "Library MCListBox Resizer.vi"("MCListbox Refnum"=w302) -> ()  [unwired: 15 in]
      }
      frame "set database" {
        n153 = property on="database" class="Ring (strict)"() -> ("Strings []"=w308:string[])  [unwired: 2 in, 2 out]
        n154 = Index Array(array=w308, index="database") -> (element=w307:string)
        n155 = Empty String/Path?(string/path=w307) -> (empty?=w309:bool)
        n156 = case shown="True" w309 {
          tunnel: w308 -> [_ w319]
          tunnel: w307 -> [w316 _]
          tunnel: [w316 w318] -> w306
          frame False {
          }
          frame True {
            w317 = 0 ("index")
            n157 = Index Array(array=w319, index=w317) -> (element=w318:string)
            n158 = local write "database"(w317) -> ()
          }
        }
      }
      frame "get subsets" {
        w333 = T8[] [enum."cleanup"] items=["empty queue", "poll list", "poll live", "resize", "set database", "get subsets", "winnow list", "filter list", "subset list", "show list", "create tag", "create meta tag", "clone tag", "rename tag", "configure tag", "chart tag", "set tag", "stat tag", "delete tag", "ablement", "initialize", "init refs", "init databases", "init persist", "cleanup", "stop"] ("Array Constant")
        w325 = "~`&%" ("string")
        n159 = local read "database infos"() -> (w342:T6)
        n160 = call "obj_ClientSrv Client Access State.vi"() -> ("certificate"=w340:string, "error out"=w343:errorcluster)  [unwired: 14 in]
        n161 = call-by-ref "?"(reference=w342, error in=w343, "method"=t_DataLog_Tag_Info_List_Methods."get subsets", "certificate in"=w340, "database (current)"=w328) -> (error out=w344:errorcluster, "subsets out"=w339:T19[], 15:"error out"=w341:errorcluster)  [unwired: 7 in, 5 out]
        n162 = local read "filter/subset"() -> (w323:string)
        n163 = call "Library Remote Call Error Merger.vi"("call by reference node error"=w344, "called VI error (no error)"=w341) -> ("error out"=w337:errorcluster)  [unwired: 13 in]
        n164 = call "Library Log Error to Window.vi"("error in (no error)"=w337) -> ("dup error"=w336:errorcluster)  [unwired: 13 in, 1 out]
        n165 = String Subset(string=w323, length (rest)=4 ("length (rest)")) -> (substring=w326:string)  [unwired: 1 in]
        n166 = Not Equal?(x=w325, y=w326) -> (x != y?=w324:bool)
        n167 = Select(t=w323, s=w324, f="") -> (s? t:f=w322:string)
        n168 = for {
          tunnel: w339 -> [w360] mode=indexing
          shift-right: [w356] -> w331
          shift-left: cluster{"String":string, "Value":string} {"String"="all tags", "Value"=""} -> [w356]
          tunnel: [w355] -> w332 mode=indexing
          shift-right: [w350] -> w320
          shift-left: w322 -> [w348]
          tunnel: w323 -> [w349]
          tunnel: w325 -> [w352]
          n169 = Unbundle By Name(w360) -> ("name"=w357:string)
          n170 = Concatenate Strings(w352, w357) -> (w353:string)
          n171 = Equal?(x=w353, y=w349) -> (x = y?=w351:bool)
          n172 = Concatenate Strings("subset \"" ("string"), w357, "\"" ("string")) -> (w354:string)
          n173 = Bundle By Name(cluster=w356, "String"=w354, "Value"=w353) -> (w355:cluster{"String":string, "Value":string})
          n174 = Select(t=w349, s=w351, f=w348) -> (s? t:f=w350:string)
        }
        n175 = Build Array (concatenate)(w331, w332) -> (w330:cluster{"String":string, "Value":string}[])
        n176 = property on="filter/subset" class="CmbBox"("Strings And Values []"=w330, "Value"=w320) -> ()  [unwired: 2 in, 2 out]
        n177 = Select(t=w333, s=w336, f=w334) -> (s? t:f=w335:T8[])
      }
      frame "winnow list" {
        n178 = String Subset(string="filter/subset", length (rest)=4 ("length (rest)")) -> (substring=w367:string)  [unwired: 1 in]
        n179 = Equal?(x=w367, y="~`&%" ("string")) -> (x = y?=w365:bool)
        n180 = Select(t=t_DataLog_Tag_Manager_States."subset list" ("states"), s=w365, f=t_DataLog_Tag_Manager_States."filter list" ("states")) -> (s? t:f=w364:T8)
        n181 = Build Array (concatenate)(w364, w374) -> (w375:T8[])
      }
      frame "filter list" {
        n182 = local read "filter/subset"() -> (w377:string)
        n183 = Array Size(array=w385) -> (size(s)=w384:i32)
        n184 = call "Library Wildcards to Regular.vi"("wildcards"=w377) -> ("regular expression"=w380:string)  [unwired: 4 in]
        n185 = for {
          N: w384 -> [_]
          shift-right: [w398] -> w381
          shift-left: i32[] [] -> [w399]
          shift-right: [w407] -> w387
          shift-left: w385 -> [w407]
          tunnel: w380 -> [w396]
          i -> [w397]
          n186 = Index Array(array=w407, index=w397) -> (element=w406:T15)
          n187 = Unbundle By Name(w406) -> ("is meta?"=w404:bool, "name"=w405:string)
          n188 = Compound Arithmetic op=OR(invert "hide meta?", invert w404) -> (w401:bool)
          n189 = Match Pattern(string=w405, regular expression=w396) -> (offset past match=w395:i32)  [unwired: 1 in, 3 out]
          n190 = Greater Or Equal To 0?(x=w395) -> (x >= 0?=w402:bool)
          n191 = And(x=w401, y=w402) -> (x .and. y?=w400:bool)
          n192 = case shown="True" w400 {
            tunnel: w399 -> [w408 w411]
            tunnel: [w408 w410] -> w398
            tunnel: w397 -> [_ w409]
            frame False {
            }
            frame True {
              n193 = Build Array (concatenate)(w411, w409) -> (w410:i32[])
            }
          }
        }
        n194 = for {
          tunnel: w381 -> [w394] mode=indexing
          shift-right: [w393] -> w386
          shift-left: w387 -> [w393]
          tunnel: [w392] -> w383 mode=indexing
          n195 = Index Array(array=w393, index=w394) -> (element=w392:T15)
        }
        n196 = Array Size(array=w381) -> (size(s)=→"shown tags":i32)
        n197 = Build Array (concatenate)(t_DataLog_Tag_Manager_States."show list" ("states"), w390) -> (w391:T8[])
      }
      frame "subset list" {
        n198 = for {
          tunnel: w416 -> [w466] mode=indexing
          tunnel: [w465] -> w418 mode=indexing
          n199 = Unbundle By Name(w466) -> ("name"=w465:string)
        }
        n200 = local read "filter/subset"() -> (w414:string)
        n201 = String Subset(string=w414, offset (0)=4) -> (substring=w417:string)  [unwired: 1 in]
        n202 = Search 1D Array(1D array=w418, element=w417) -> (index of element=w415:i32)  [unwired: 1 in]
        n203 = Less Than 0?(x=w415) -> (x < 0?=w413:bool)
        n204 = case "selected subset no longer present?" shown="False" w413 {
          tunnel: [w439 w464] -> w423
          tunnel: w422 -> [w438 w464]
          tunnel: [w436 w464] -> w421
          tunnel: w416 -> [w433 _]
          tunnel: w415 -> [w430 _]
          frame False {
            # "avoid LV7 bug"
            n205 = Index Array(array=w433, index=w430) -> (element=w432:T19)
            n206 = Array Size(array=w438) -> (size(s)=w437:i32)
            n207 = Unbundle By Name(w432) -> ("tags"=w431:string[])
            n208 = for {
              N: w437 -> [_]
              shift-right: [w453] -> w435
              shift-left: cluster{"index of element":i32, i32}[] [] -> [w454]
              shift-right: [w458] -> w440
              shift-left: w438 -> [w458]
              tunnel: w431 -> [w450]
              i -> [w446]
              n209 = Index Array(array=w458, index=w446) -> (element=w457:T15)
              n210 = local read "hide meta?"() -> (w452:bool)
              n211 = Unbundle By Name(w457) -> ("is meta?"=w456:bool, "name"=w451:string)
              n212 = Search 1D Array(1D array=w450, element=w451) -> (index of element=w447:i32)  [unwired: 1 in]
              n213 = Compound Arithmetic op=OR(invert w452, invert w456) -> (w455:bool)
              n214 = Greater Or Equal To 0?(x=w447) -> (x >= 0?=w448:bool)
              n215 = Bundle("index of element"=w447, w446) -> (w445:cluster{"index of element":i32, i32})  [unwired: 1 in]
              n216 = And(x=w455, y=w448) -> (x .and. y?=w449:bool)
              n217 = case shown="True" w449 {
                tunnel: w454 -> [w459 w460]
                tunnel: [w459 w462] -> w453
                tunnel: w445 -> [_ w461]
                frame False {
                }
                frame True {
                  n218 = Build Array (concatenate)(w460, w461) -> (w462:cluster{"index of element":i32, i32}[])
                }
              }
            }
            n219 = Sort 1D Array(array=w435) -> (sorted array=w428:cluster{"index of element":i32, i32}[])
            n220 = Array Size(array=w435) -> (size(s)=w434:i32)
            n221 = Sort 1D Array(array=w428) -> (sorted array=w427:cluster{"index of element":i32, i32}[])
            n222 = local write "shown tags"(w434) -> ()
            n223 = for {
              tunnel: w427 -> [w442] mode=indexing
              shift-right: [w444] -> w439
              shift-left: w440 -> [w444]
              tunnel: [w443] -> w436 mode=indexing
              n224 = Unbundle(w442) -> (w441:i32)  [unwired: 1 out]
              n225 = Index Array(array=w444, index=w441) -> (element=w443:T15)
            }
          }
          frame True {
            n226 = local write "filter/subset"("") -> ()
          }
        }
        n227 = Build Array (concatenate)(t_DataLog_Tag_Manager_States."show list" ("states"), w425) -> (w426:T8[])
      }
      frame "show list" {
        n228 = stacked-sequence {
          tunnel: w470 -> [w482 _]
          frame #0 {
            n229 = To Lower Case(string="selected") -> (all lower case string=w479:string)
            n230 = for {
              tunnel: w482 -> [w505] mode=indexing
              tunnel: [w504] -> w483 mode=indexing
              shift-right: [w497] -> _
              shift-left: FALSE -> [w495]
              tunnel: w479 -> [w494]
              i -> [w496]
              # "Sort order is case  insensitive.\nSet selection to same tag or\nfirst tag after when the\nselected tag has disappeared."
              n231 = Unbundle By Name(w505) -> ("name"=w487:string, "value"=w486:T13, "unit"=w484:string, "logging algorithm"=w503:T17, "description"=w500:string, "expression"=w492:string, "update"=w491:bool, "temporal"=w502:T12)
              n232 = To Lower Case(string=w487) -> (all lower case string=w493:string)
              n233 = case shown="\"string\"" w486 {
                tunnel: ["<number>" "<string>"] -> w485
                frame "number", Default {
                }
                frame "string" {
                }
              }
              n234 = Format Into String(w503) -> (resulting string=w488:string)  [unwired: 3 in, 1 out]
              n235 = Format Into String(w502) -> (resulting string=w501:string)  [unwired: 3 in, 1 out]
              n236 = Greater?(x=w494, y=w493) -> (0:w499:bool)
              n237 = Or(x=w495, y=w499) -> (x .or. y?=w498:bool)
              n238 = Select(t=w492, s=w491, f="") -> (s? t:f=w489:string)
              n239 = case shown="False" w498 {
                tunnel: [TRUE w511] -> w497
                tunnel: w496 -> [w510 _]
                tunnel: w487 -> [w509 _]
                tunnel: w495 -> [_ w511]
                frame False {
                  n240 = local write "selected"(w509) -> ()
                  n241 = local write "tag list"(w510) -> ()
                }
                frame True {
                }
              }
              n242 = Build Array(w487, w485, w484, w488, w489, w500, w501) -> (w504:string[])
            }
            n243 = property on="tag list" class="MCListbox (strict)"("Item Names"=w483, "Active Cell:Active Cell"=cluster{i32, i32} {-2, -2} ("Active Cell"), "Active Cell:Cell Background Color"=u32 15790320, "Active Cell:Active Cell"=cluster{i32, i32} {-1, -2} ("Active Cell"), "Active Cell:Cell Background Color"=u32 11776947) -> ()  [unwired: 2 in, 2 out]
          }
          frame #1 {
            n244 = property on="tag list" class="MCListbox (strict)"() -> ("Number of Rows"=w514:u32, "Top Left Visible Cell"=w512:T18)  [unwired: 2 in, 2 out]
            n245 = Unbundle(w512) -> ("Row"=w518:u32)  [unwired: 1 out]
            n246 = Add(x=w514, y=w518) -> (x+y=w519:u32)
            n247 = To Long Integer(number=w519) -> (32bit integer=w513:i32)
            n248 = To Long Integer(number=w518) -> (32bit integer=w517:i32)
            n249 = local read "tag list"() -> (w515:i32)
            n250 = In Range and Coerce(upper limit=w513, x=w515, lower limit=w517) -> (In Range?=w516:bool)  [unwired: 1 out]
            n251 = case shown="False" w516 {
              tunnel: w515 -> [w529 _]
              tunnel: w513 -> [w528 _]
              tunnel: w512 -> [w523 _]
              frame False {
                n252 = Quotient & Remainder(x=w528, y=2) -> (floor(x/y)=w526:i32)  [unwired: 1 out]
                n253 = Subtract(x=w529, y=w526) -> (x-y=w525:i32)
                n254 = Max & Min(x=w525, y=0) -> (max(x,y)=w522:i32)  [unwired: 1 out]
                n255 = To Unsigned Long Integer(number=w522) -> (unsigned 32bit integer=w521:u32)
                n256 = Bundle(cluster=w523, "Row"=w521) -> (w520:T18)  [unwired: 1 in]
                n257 = property on="tag list" class="MCListbox (strict)"("Top Left Visible Cell"=w520) -> ()  [unwired: 2 in, 2 out]
              }
              frame True {
              }
            }
          }
        }
        n258 = Build Array (concatenate)(t_DataLog_Tag_Manager_States."ablement" ("states"), w473) -> (w474:T8[])
      }
      frame "create tag" {
        n259 = call "ui_Library Query String.vi"("prompt"="Enter the name of the tag to create.") -> ("OKed?"=w537:bool, "string out"=w538:string)  [unwired: 13 in]
        n260 = case "OKed?" shown="True" w537 {
          tunnel: w538 -> [_ w555]
          tunnel: [w540 w558] -> w535
          tunnel: w534 -> [w540 w557]
          tunnel: w532 -> [_ w541]
          frame False {
          }
          frame True {
            n261 = local read "database infos"() -> (w542:T6)
            n262 = call "obj_ClientSrv Client Access State.vi"() -> ("certificate"=w543:string, "error out"=w554:errorcluster)  [unwired: 14 in]
            n263 = call-by-ref "?"(reference=w542, error in=w554, "method"=t_DataLog_Tag_Info_List_Methods."test tag", "tag or base tag"=w555, "certificate in"=w543, "database (current)"=w541) -> (reference out=w544:T6, error out=w553:errorcluster, 15:"error out"=w552:errorcluster)  [unwired: 6 in, 5 out]
            n264 = call "Library Remote Call Error Merger.vi"("call by reference node error"=w553, "called VI error (no error)"=w552) -> ("error out"=w549:errorcluster)  [unwired: 13 in]
            n265 = call-by-ref "?"(reference=w544, error in=w549, "method"=t_DataLog_Tag_Info_List_Methods."get default", "certificate in"=w543, "database (current)"=w541) -> (reference out=w545:T6, error out=w551:errorcluster, "tag config out"=w546:T15, 15:"error out"=w548:errorcluster)  [unwired: 7 in, 4 out]
            n266 = call "Library Remote Call Error Merger.vi"("call by reference node error"=w551, "called VI error (no error)"=w548) -> ("error out"=w547:errorcluster)  [unwired: 13 in]
            n267 = case shown="No Error" w547 {
              selector: w547 -> [_ w590]
              tunnel: w545 -> [w568 _]
              tunnel: w555 -> [w566 _]
              tunnel: [w563 w589] -> w558
              tunnel: w557 -> [w562 w589]
              tunnel: w541 -> [w561 _]
              tunnel: w546 -> [w560 _]
              frame No Error {
                n268 = call "ui_DataLog Query Tag Creation Parameters.vi"("default config"=w560) -> ("initial value out"=w564:dbl, "OKed?"=w565:bool, "info out"=w567:T15, "initial string out"=w559:string)  [unwired: 11 in]
                n269 = case "OKed?" shown="True" w565 {
                  tunnel: w568 -> [_ w584]
                  tunnel: w567 -> [_ w578]
                  tunnel: w566 -> [_ w581]
                  tunnel: w564 -> [_ w579]
                  tunnel: [w569 w583] -> w563
                  tunnel: w562 -> [w569 w582]
                  tunnel: w561 -> [_ w571]
                  tunnel: w559 -> [_ w570]
                  frame False {
                  }
                  frame True {
                    n270 = call "obj_ClientSrv Client Access State.vi"("access level (observer)"=t_ClientSrv_Access_Levels."operator") -> ("certificate"=w572:string, "error out"=w574:errorcluster)  [unwired: 13 in]
                    n271 = call-by-ref "?"(reference=w584, error in=w574, "method"=t_DataLog_Tag_Info_List_Methods."create", "initial number (NaN)"=w579, "tag or base tag"=w581, "tag config in"=w578, "certificate in"=w572, "initial string (\"\")"=w570, "database (current)"=w571) -> (error out=w577:errorcluster, 15:"error out"=w576:errorcluster)  [unwired: 3 in, 6 out]
                    n272 = call "Library Remote Call Error Merger.vi"("call by reference node error"=w577, "called VI error (no error)"=w576) -> ("error out"=w575:errorcluster)  [unwired: 13 in]
                    n273 = case shown="No Error" w575 {
                      selector: w575 -> [_ w587]
                      tunnel: w581 -> [w586 _]
                      tunnel: [w585 w588] -> w583
                      tunnel: w582 -> [_ w588]
                      frame No Error {
                        w585 = T8[] [enum."poll list", enum."configure tag"] items=["empty queue", "poll list", "poll live", "resize", "set database", "get subsets", "winnow list", "filter list", "subset list", "show list", "create tag", "create meta tag", "clone tag", "rename tag", "configure tag", "chart tag", "set tag", "stat tag", "delete tag", "ablement", "initialize", "init refs", "init databases", "init persist", "cleanup", "stop"] ("Array Constant")
                        n274 = local write "selected"(w586) -> ()
                      }
                      frame Error {
                        n275 = call "Library Log Error to Window.vi"("error in (no error)"=w587) -> ()  [unwired: 13 in, 2 out]
                      }
                    }
                  }
                }
              }
              frame Error {
                n276 = call "Library Log Error to Window.vi"("error in (no error)"=w590) -> ()  [unwired: 13 in, 2 out]
              }
            }
          }
        }
      }
      frame "create meta tag" {
        n277 = local read "tag list"() -> (w597:i32)
        n278 = Index Array(array=w601, index=w597) -> (element=w600:T15)
        n279 = Unbundle By Name(w600) -> ("name"=w593:string)
        n280 = call "ui_DataLog Query Meta.vi"("base tag"=w593) -> ("initial value out"=w596:dbl, "OKed?"=w602:bool, "meta out"=w603:T7)  [unwired: 12 in]
        n281 = case "OKed?" shown="True" w602 {
          tunnel: w603 -> [_ w606]
          tunnel: w593 -> [_ w605]
          tunnel: [w604 w626] -> w599
          tunnel: w598 -> [w604 w625]
          tunnel: w596 -> [_ w624]
          tunnel: w594 -> [_ w607]
          frame False {
          }
          frame True {
            n282 = local read "database infos"() -> (w608:T6)
            n283 = call "obj_ClientSrv Client Access State.vi"() -> ("certificate"=w610:string, "error out"=w609:errorcluster)  [unwired: 14 in]
            n284 = call-by-ref "?"(reference=w608, error in=w609, "method"=t_DataLog_Tag_Info_List_Methods."get default", "tag or base tag"=w605, "certificate in"=w610, "database (current)"=w607) -> (reference out=w613:T6, error out=w614:errorcluster, "tag config out"=w612:T15, 15:"error out"=w616:errorcluster)  [unwired: 6 in, 4 out]
            n285 = call "Library Remote Call Error Merger.vi"("call by reference node error"=w614, "called VI error (no error)"=w616) -> ("error out"=w611:errorcluster)  [unwired: 13 in]
            n286 = call "obj_ClientSrv Client Access State.vi"("access level (observer)"=t_ClientSrv_Access_Levels."operator", "error in (no error)"=w611) -> ("certificate"=w617:string, "error out"=w619:errorcluster)  [unwired: 12 in]
            n287 = call-by-ref "?"(reference=w613, error in=w619, "method"=t_DataLog_Tag_Info_List_Methods."create", "initial number (NaN)"=w624, "tag or base tag"=w605, "tag config in"=w612, "meta specifier (not a meta)"=w606, "certificate in"=w617, "database (current)"=w607) -> (error out=w622:errorcluster, 15:"error out"=w621:errorcluster)  [unwired: 3 in, 6 out]
            n288 = call "Library Remote Call Error Merger.vi"("call by reference node error"=w622, "called VI error (no error)"=w621) -> ("error out"=w620:errorcluster)  [unwired: 13 in]
            n289 = case shown="No Error" w620 {
              selector: w620 -> [_ w631]
              tunnel: [w630 w632] -> w626
              tunnel: w625 -> [_ w632]
              tunnel: w606 -> [w628 _]
              tunnel: w605 -> [w627 _]
              frame No Error {
                w630 = T8[] [enum."poll list", enum."configure tag"] items=["empty queue", "poll list", "poll live", "resize", "set database", "get subsets", "winnow list", "filter list", "subset list", "show list", "create tag", "create meta tag", "clone tag", "rename tag", "configure tag", "chart tag", "set tag", "stat tag", "delete tag", "ablement", "initialize", "init refs", "init databases", "init persist", "cleanup", "stop"] ("Array Constant")
                n290 = call "DataLog Append Meta Specifier.vi"("meta specifier"=w628, "tag in"=w627) -> ("tag out"=w629:string)  [unwired: 13 in]
                n291 = local write "selected"(w629) -> ()
              }
              frame Error {
                n292 = call "Library Log Error to Window.vi"("error in (no error)"=w631) -> ()  [unwired: 13 in, 2 out]
              }
            }
          }
        }
      }
      frame "clone tag" {
        n293 = local read "tag list"() -> (w639:i32)
        n294 = Index Array(array=w638, index=w639) -> (element=w636:T15)
        n295 = Unbundle By Name(w636) -> ("name"=w637:string)
        n296 = call "ui_Library Query String.vi"("prompt"="Enter the name of the cloned tag.", "string in (\"\")"=w637) -> ("OKed?"=w644:bool, "string out"=w645:string)  [unwired: 12 in]
        n297 = case "OKed?" shown="True" w644 {
          tunnel: w645 -> [_ w657]
          tunnel: [w646 w658] -> w642
          tunnel: w641 -> [w646 _]
          tunnel: w636 -> [_ w656]
          tunnel: w635 -> [_ w647]
          frame False {
          }
          frame True {
            w658 = T8[] [enum."poll list"] items=["empty queue", "poll list", "poll live", "resize", "set database", "get subsets", "winnow list", "filter list", "subset list", "show list", "create tag", "create meta tag", "clone tag", "rename tag", "configure tag", "chart tag", "set tag", "stat tag", "delete tag", "ablement", "initialize", "init refs", "init databases", "init persist", "cleanup", "stop"] ("Array Constant")
            n298 = local read "database infos"() -> (w649:T6)
            n299 = call "obj_ClientSrv Client Access State.vi"("access level (observer)"=t_ClientSrv_Access_Levels."operator") -> ("certificate"=w648:string, "error out"=w650:errorcluster)  [unwired: 13 in]
            n300 = call-by-ref "?"(reference=w649, error in=w650, "method"=t_DataLog_Tag_Info_List_Methods."create", "tag or base tag"=w657, "tag config in"=w656, "certificate in"=w648, "database (current)"=w647) -> (error out=w654:errorcluster, 15:"error out"=w653:errorcluster)  [unwired: 5 in, 6 out]
            n301 = call "Library Remote Call Error Merger.vi"("call by reference node error"=w654, "called VI error (no error)"=w653) -> ("error out"=w652:errorcluster)  [unwired: 13 in]
            n302 = case shown="No Error" w652 {
              selector: w652 -> [_ w660]
              tunnel: w657 -> [w659 _]
              frame No Error {
                n303 = local write "selected"(w659) -> ()
              }
              frame Error {
                n304 = call "Library Log Error to Window.vi"("error in (no error)"=w660) -> ()  [unwired: 13 in, 2 out]
              }
            }
          }
        }
      }
      frame "rename tag" {
        n305 = local read "tag list"() -> (w673:i32)
        n306 = Index Array(array=w674, index=w673) -> (element=w668:T15)
        n307 = Unbundle By Name(w668) -> ("name"=w665:string)
        n308 = Format Into String(format string="Enter a new name for tag \"%s\"" ("prompt"), w665) -> (resulting string=w666:string)  [unwired: 2 in, 1 out]
        n309 = call "ui_Library Query String.vi"("prompt"=w666, "string in (\"\")"=w665) -> ("OKed?"=w669:bool, "string out"=w670:string)  [unwired: 12 in]
        n310 = case "OKed?" shown="True" w669 {
          tunnel: [w675 w687] -> w672
          tunnel: w671 -> [w675 _]
          tunnel: w668 -> [_ w686]
          tunnel: w670 -> [_ w685]
          tunnel: w663 -> [_ w676]
          frame False {
          }
          frame True {
            w687 = T8[] [enum."poll list"] items=["empty queue", "poll list", "poll live", "resize", "set database", "get subsets", "winnow list", "filter list", "subset list", "show list", "create tag", "create meta tag", "clone tag", "rename tag", "configure tag", "chart tag", "set tag", "stat tag", "delete tag", "ablement", "initialize", "init refs", "init databases", "init persist", "cleanup", "stop"] ("Array Constant")
            n311 = call "obj_ClientSrv Client Access State.vi"("access level (observer)"=t_ClientSrv_Access_Levels."operator") -> ("certificate"=w677:string, "error out"=w679:errorcluster)  [unwired: 13 in]
            n312 = local read "database infos"() -> (w678:T6)
            n313 = call-by-ref "?"(reference=w678, error in=w679, "method"=t_DataLog_Tag_Info_List_Methods."rename", "tag or base tag"=w685, "tag config in"=w686, "certificate in"=w677, "database (current)"=w676) -> (error out=w682:errorcluster, 15:"error out"=w683:errorcluster)  [unwired: 5 in, 6 out]
            n314 = call "Library Remote Call Error Merger.vi"("call by reference node error"=w682, "called VI error (no error)"=w683) -> ("error out"=w681:errorcluster)  [unwired: 13 in]
            n315 = case shown="Error" w681 {
              selector: w681 -> [_ w689]
              tunnel: w685 -> [w688 _]
              frame No Error {
                n316 = local write "selected"(w688) -> ()
              }
              frame Error {
                n317 = call "Library Log Error to Window.vi"("error in (no error)"=w689) -> ()  [unwired: 13 in, 2 out]
              }
            }
          }
        }
      }
      frame "configure tag" {
        n318 = local read "tag list"() -> (w696:i32)
        n319 = Index Array(array=w697, index=w696) -> (element=w693:T15)
        n320 = while "while OKed but not OK" {
          tunnel: [w702] -> w694
          shift-right: [w699] -> _
          shift-left: w693 -> [w700]
          tunnel: w692 -> [w698]
          stop <- w701 continue-if-true
          n321 = call "ui_DataLog Query Tag Configuration.vi"("info in"=w700) -> ("OKed?"=w703:bool, "info out"=w704:T15)  [unwired: 13 in]
          n322 = case "OKed?" shown="True" w703 {
            tunnel: w704 -> [w705 w707]
            tunnel: [_ w717] -> w702
            tunnel: [_ w710] -> w701
            tunnel: [w705 w707] -> w699
            tunnel: w698 -> [_ w709]
            frame False {
            }
            frame True {
              w717 = T8[] [enum."poll list"] items=["empty queue", "poll list", "poll live", "resize", "set database", "get subsets", "winnow list", "filter list", "subset list", "show list", "create tag", "create meta tag", "clone tag", "rename tag", "configure tag", "chart tag", "set tag", "stat tag", "delete tag", "ablement", "initialize", "init refs", "init databases", "init persist", "cleanup", "stop"] ("Array Constant")
              n323 = Unbundle By Name(w707) -> ("name"=w706:string)
              n324 = call "obj_ClientSrv Client Access State.vi"("access level (observer)"=t_ClientSrv_Access_Levels."operator") -> ("certificate"=w708:string, "error out"=w714:errorcluster)  [unwired: 13 in]
              n325 = local read "database infos"() -> (w713:T6)
              n326 = call-by-ref "?"(reference=w713, error in=w714, "method"=t_DataLog_Tag_Info_List_Methods."set config", "tag or base tag"=w706, "tag config in"=w707, "certificate in"=w708, "database (current)"=w709) -> (error out=w716:errorcluster, 15:"error out"=w711:errorcluster)  [unwired: 5 in, 6 out]
              n327 = case shown="Error" w711 {
                selector: w711 -> [_ w724]
                tunnel: [_ w720] -> w710
                frame No Error {
                }
                frame Error {
                  n328 = call "Library Explain Error.vi"("explanation prefix (none)"="Cannot set configuration.", "error in (no error)"=w724) -> ("explained error"=w722:errorcluster)  [unwired: 13 in]
                  n329 = Unbundle By Name(w722) -> ("source"=w721:string)
                  n330 = Two Button Dialog(message=w721, 2:"Let me fix it" ("T button name (\"OK\")")) -> (T button?=w720:bool)  [unwired: 1 in]
                }
              }
              n331 = call "Library Remote Call Error Merger.vi"("call by reference node error"=w716) -> ("error out"=w712:errorcluster)  [unwired: 14 in]
              n332 = call "Library Log Error to Window.vi"("error in (no error)"=w712) -> ()  [unwired: 13 in, 2 out]
            }
          }
        }
      }
      frame "chart tag" {
        n333 = local read "tag list"() -> (w736:i32)
        n334 = Index Array(array=w737, index=w736) -> (element=w733:T15)
        n335 = Unbundle By Name(w733) -> ("name"=w732:string)
        n336 = call "Library Resolve VI Path.vi"("VI name"="tui_DataLog Live Tag Chart.vit") -> ("VI path"=w729:path)  [unwired: 14 in]
        n337 = call "obj_Library Session.vi"("method"=t_Library_Session_Methods."run", "path"=w729, "argument in (none)"=w732) -> ("error out"=w730:errorcluster)  [unwired: 9 in, 3 out]
        n338 = call "Library Log Error to Window.vi"("error in (no error)"=w730) -> ()  [unwired: 13 in, 2 out]
      }
      frame "set tag" {
        w746 = T8[] [enum."poll live"] items=["empty queue", "poll list", "poll live", "resize", "set database", "get subsets", "winnow list", "filter list", "subset list", "show list", "create tag", "create meta tag", "clone tag", "rename tag", "configure tag", "chart tag", "set tag", "stat tag", "delete tag", "ablement", "initialize", "init refs", "init databases", "init persist", "cleanup", "stop"] ("Array Constant")
        n339 = local read "tag list"() -> (w749:i32)
        n340 = Index Array(array=w750, index=w749) -> (element=w740:T15)
        n341 = call "ui_DataLog Query New Value.vi"("tag info"=w740) -> ("OKed?"=w743:bool, "new value out"=w741:dbl)  [unwired: 13 in]
        n342 = case "OKed?" shown="True" w743 {
          selector: w743 -> [w751 w762]
          tunnel: [w751 w762] -> w742
          tunnel: w741 -> [_ w758]
          tunnel: w740 -> [_ w757]
          frame False {
          }
          frame True {
            n343 = Unbundle By Name(w757) -> ("name"=w756:string)
            n344 = call "obj_ClientSrv Client Access State.vi"("access level (observer)"=t_ClientSrv_Access_Levels."operator") -> ("certificate"=w753:string, "error out"=w752:errorcluster)  [unwired: 13 in]
            n345 = local read "set tag value"() -> (w759:T2)
            n346 = call-by-ref "?"(reference=w759, error in=w752, "tag"=w756, "value"=w758, "certificate"=w753) -> (error out=w761:errorcluster, 15:"error out"=w760:errorcluster)  [unwired: 12 in, 1 out]
            n347 = call "Library Remote Call Error Merger.vi"("call by reference node error"=w761, "called VI error (no error)"=w760) -> ("error out"=w755:errorcluster)  [unwired: 13 in]
            n348 = call "Library Log Error to Window.vi"("error in (no error)"=w755) -> ()  [unwired: 13 in, 2 out]
          }
        }
        n349 = Select(t=w746, s=w742, f=w745) -> (s? t:f=w747:T8[])
      }
      frame "stat tag" {
        n350 = local read "tag list"() -> (w777:i32)
        n351 = Index Array(array=w778, index=w777) -> (element=w765:T15)
        n352 = Unbundle By Name(w765) -> ("name"=w770:string)
        n353 = call "obj_ClientSrv Client Access State.vi"() -> ("certificate"=w769:string, "error out"=w768:errorcluster)  [unwired: 14 in]
        n354 = local read "dump tag buffer"() -> (w771:T1)
        n355 = call-by-ref "?"(reference=w771, error in=w768, "certificate"=w769, "tag"=w770) -> (error out=w773:errorcluster, "points"=w766:T20[], 15:"error out"=w772:errorcluster)  [unwired: 12 in, 1 out]
        n356 = call "Library Remote Call Error Merger.vi"("call by reference node error"=w773, "called VI error (no error)"=w772) -> ("error out"=w767:errorcluster)  [unwired: 13 in]
        n357 = case shown="No Error" w767 {
          selector: w767 -> [_ w782]
          tunnel: w766 -> [w781 _]
          tunnel: w765 -> [w780 _]
          frame No Error {
            n358 = call "DataLog Format Stats.vi"("tag config"=w780, "points"=w781) -> ("stats"=w779:string)
            n359 = One Button Dialog(message=w779) -> ()  [unwired: 1 in, 1 out]
          }
          frame Error {
            n360 = call "Library Log Error to Window.vi"("error in (no error)"=w782) -> ()  [unwired: 13 in, 2 out]
          }
        }
      }
      frame "delete tag" {
        n361 = local read "tag list"() -> (w796:i32)
        n362 = Index Array(array=w797, index=w796) -> (element=w793:T15)
        n363 = Unbundle By Name(w793) -> ("name"=w785:string)
        n364 = Format Into String(format string="Are you sure that tag \"%s\"\nand all its logged data must be deleted?" ("prompt"), w785) -> (resulting string=w791:string)  [unwired: 2 in, 1 out]
        n365 = Two Button Dialog(message=w791, 1:"No" ("F button name (\"Cancel\")"), 2:"Yes" ("T button name (\"OK\")")) -> (T button?=w788:bool)
        n366 = case "OKed?" shown="True" w788 {
          tunnel: [w798 w809] -> w795
          tunnel: w794 -> [w798 _]
          tunnel: w786 -> [_ w801]
          tunnel: w785 -> [_ w799]
          frame False {
          }
          frame True {
            w809 = T8[] [enum."poll list"] items=["empty queue", "poll list", "poll live", "resize", "set database", "get subsets", "winnow list", "filter list", "subset list", "show list", "create tag", "create meta tag", "clone tag", "rename tag", "configure tag", "chart tag", "set tag", "stat tag", "delete tag", "ablement", "initialize", "init refs", "init databases", "init persist", "cleanup", "stop"] ("Array Constant")
            n367 = call "obj_ClientSrv Client Access State.vi"("access level (observer)"=t_ClientSrv_Access_Levels."operator") -> ("certificate"=w800:string, "error out"=w804:errorcluster)  [unwired: 13 in]
            n368 = local read "database infos"() -> (w802:T6)
            n369 = call-by-ref "?"(reference=w802, error in=w804, "method"=t_DataLog_Tag_Info_List_Methods."delete", "tag or base tag"=w799, "certificate in"=w800, "database (current)"=w801) -> (error out=w807:errorcluster, 15:"error out"=w806:errorcluster)  [unwired: 6 in, 6 out]
            n370 = call "Library Remote Call Error Merger.vi"("call by reference node error"=w807, "called VI error (no error)"=w806) -> ("error out"=w805:errorcluster)  [unwired: 13 in]
            n371 = call "Library Log Error to Window.vi"("error in (no error)"=w805) -> ()  [unwired: 13 in, 2 out]
          }
        }
      }
      frame "ablement" {
        w816 = u8 2 items=["enabled", "disabled", "grayed"] ("disabled state")
        n372 = local read "mode"() -> (w817:T3)
        n373 = case shown="\"mirrored\"" w817 {
          tunnel: [w847 w851 w854 w857] -> w813
          tunnel: [w845 w850 w852 w855] -> w815
          tunnel: [w846 w849 w853 w856] -> w814
          tunnel: [w845 w848 w852 w855] -> w810
          frame "locked" {
            w846 = u8 2 items=["enabled", "disabled", "grayed"] ("disabled state")
            w845 = u8 2 items=["enabled", "disabled", "grayed"] ("disabled state")
            w847 = u8 2 items=["enabled", "disabled", "grayed"] ("disabled state")
          }
          frame "mirrored" {
            w848 = u8 0 items=["enabled", "disabled", "grayed"] ("disabled state")
            w849 = u8 2 items=["enabled", "disabled", "grayed"] ("disabled state")
            w850 = u8 2 items=["enabled", "disabled", "grayed"] ("disabled state")
            w851 = u8 2 items=["enabled", "disabled", "grayed"] ("disabled state")
          }
          frame "unlocked" {
            w853 = u8 0 items=["enabled", "disabled", "grayed"] ("disabled state")
            w852 = u8 0 items=["enabled", "disabled", "grayed"] ("disabled state")
            w854 = u8 2 items=["enabled", "disabled", "grayed"] ("disabled state")
          }
          frame "live" {
            w856 = u8 0 items=["enabled", "disabled", "grayed"] ("disabled state")
            w855 = u8 2 items=["enabled", "disabled", "grayed"] ("disabled state")
            w857 = u8 0 items=["enabled", "disabled", "grayed"] ("disabled state")
          }
        }
        n374 = Index Array(array=w840, index="tag list") -> (element=w843:T15)
        n375 = Array Size(array=w840) -> (size(s)=w839:i32)
        n376 = Unbundle By Name(w843) -> ("value"=w826:T13, "is meta?"=w834:bool, "name"=w841:string, "temporal"=w824:T12)
        n377 = Equal To 0?(x=w839) -> (x = 0?=w836:bool)
        n378 = In Range and Coerce(upper limit=w839, x="tag list", lower limit=0) -> (In Range?=w835:bool)  [unwired: 1 out]
        n379 = property on="stats" class="Bool"("Disabled"=w813) -> ()  [unwired: 2 in, 2 out]
        n380 = Compound Arithmetic op=OR(w836, invert w835) -> (w830:bool)
        n381 = Not Equal?(x=w824, y=t_DataLog_Temporal_Types."set&hold" ("temporal")) -> (x != y?=w819:bool)
        n382 = Equal?(x=t_DataLog_Value_Types."string" ("valuation"), y=w826) -> (x = y?=w820:bool)
        n383 = local write "selected"(w841) -> ()
        n384 = Or(x=w830, y=w834) -> (x .or. y?=w833:bool)
        n385 = Or(x=w819, y=w820) -> (x .or. y?=w821:bool)
        n386 = Select(t=w816, s=w833, f=w815) -> (s? t:f=w829:u8)
        n387 = Select(t=w816, s=w830, f=w810) -> (s? t:f=w832:u8)
        n388 = Select(t=w816, s=w830, f=w814) -> (s? t:f=w831:u8)
        n389 = Select(t=w816, s=w821, f=w813) -> (s? t:f=w822:u8)
        n390 = Select(t=w816, s=w820, f=w813) -> (s? t:f=w825:u8)
        n391 = property on="set" class="Bool"("Disabled"=w822) -> ()  [unwired: 2 in, 2 out]
        n392 = property on="chart" class="Bool"("Disabled"=w825) -> ()  [unwired: 2 in, 2 out]
        n393 = property on="create" class="Bool"("Disabled"=w815) -> ()  [unwired: 2 in, 2 out]
        n394 = property on="delete" class="Bool"("Disabled"=w832) -> ()  [unwired: 2 in, 2 out]
        n395 = property on="configure" class="Bool"("Disabled"=w831) -> ()  [unwired: 2 in, 2 out]
        n396 = property on="clone" class="Bool"("Disabled"=w829) -> ()  [unwired: 2 in, 2 out]
        n397 = property on="rename" class="Bool"("Disabled"=w829) -> ()  [unwired: 2 in, 2 out]
        n398 = Select(t=w816, s=w820, f=w829) -> (s? t:f=w828:u8)
        n399 = property on="create meta" class="Bool"("Disabled"=w828) -> ()  [unwired: 2 in, 2 out]
      }
      frame "initialize" {
        n400 = while "rebuild init list on first run or after load or recompile" {
          shift-left: _ -> [w866]
          shift-right: [w865] -> w859
          stop <- FALSE continue-if-true
          n401 = Array Size(array=w866) -> (size(s)=w867:i32)
          n402 = case shown="0" w867 {
            tunnel: [w868 w888] -> w865
            tunnel: w866 -> [w869 w888]
            frame 0 {
              n403 = while {
                shift-left: w869 -> [w878]
                shift-right: [w876] -> w868
                shift-left: _ -> [w880]
                shift-right: [w875] -> _
                i -> [w883]
                stop <- w871 continue-if-true
                n404 = To Unsigned Word Integer(number=w883) -> (unsigned 16bit integer=w881:u16)
                n405 = Type Cast(type=t_DataLog_Tag_Manager_States."initialize" ("states"), x=w881) -> (*(type *) &x=w877:T8)
                n406 = Format Into String(format string="%s" ("Format String"), w877) -> (resulting string=w875:string)  [unwired: 2 in, 1 out]
                n407 = Not Equal?(x=w875, y=w880) -> (x != y?=w871:bool)
                n408 = Match Pattern(string=w875, regular expression="^init ") -> (offset past match=w873:i32)  [unwired: 1 in, 3 out]
                n409 = Greater Or Equal To 0?(x=w873) -> (x >= 0?=w872:bool)
                n410 = And(x=w872, y=w871) -> (x .and. y?=w870:bool)
                n411 = case shown="True" w870 {
                  tunnel: w878 -> [w884 w887]
                  tunnel: w877 -> [_ w886]
                  tunnel: [w884 w885] -> w876
                  frame False {
                  }
                  frame True {
                    n412 = Build Array (concatenate)(w887, w886) -> (w885:T8[])
                  }
                }
              }
            }
            frame Default {
            }
          }
        }
      }
      frame "init refs" {
        w936 = T8[] [enum."cleanup"] items=["empty queue", "poll list", "poll live", "resize", "set database", "get subsets", "winnow list", "filter list", "subset list", "show list", "create tag", "create meta tag", "clone tag", "rename tag", "configure tag", "chart tag", "set tag", "stat tag", "delete tag", "ablement", "initialize", "init refs", "init databases", "init persist", "cleanup", "stop"] ("Array Constant")
        n413 = call "obj_ClientSrv Connection State.vi"("machine{connect}/VI{get state} name (local/no path resolution)"="DataLog Databases_srv.vi") -> ("server app ref"=w903:refnum<vi>, "resolved server path"=w902:path, "error out"=w901:errorcluster)  [unwired: 7 in, 5 out]
        n414 = local read "databases"() -> (w905:T4)
        n415 = stacked-sequence {
          tunnel: [w985] -> w904
          tunnel: [w984] -> w906
          tunnel: w901 -> [w983]
          tunnel: w903 -> [w982]
          tunnel: w902 -> [w981]
          tunnel: w905 -> [w980]
          frame #0 {
            # "avoid LV8 complaints"
            n416 = Path to Array of Strings(0:w981) -> (2:w986:string[])  [unwired: 1 out]
            n417 = Array Size(array=w986) -> (size(s)=w987:i32)
            n418 = case shown="1" w987 {
              tunnel: w981 -> [w994 w1000]
              tunnel: w982 -> [w992 w999]
              tunnel: [w990 w995] -> w985
              tunnel: [w988 w998] -> w984
              tunnel: w980 -> [w989 w997]
              tunnel: w983 -> [w991 w996]
              frame 1 {
                n419 = Path To String(path=w994) -> (string=w993:string)
                n420 = Open VI Reference(type specifier VI Refnum (for type only)=w989, application reference (local)=w992, vi path=w993, error in (no error)=w991) -> (vi reference=w990:T4, error out=w988:errorcluster)  [unwired: 2 in]
              }
              frame Default {
                n421 = Open VI Reference(type specifier VI Refnum (for type only)=w997, application reference (local)=w999, vi path=w1000, error in (no error)=w996) -> (vi reference=w995:T4, error out=w998:errorcluster)  [unwired: 2 in]
              }
            }
          }
        }
        "databases" <- w904
        n422 = local read "database infos"() -> (w917:T6)
        n423 = call "Library Open VI Ref Error Clarifier.vi"("VI path"=w902, "called VI error (no error)"=w906) -> ("error out"=w924:errorcluster)  [unwired: 13 in]
        n424 = call "obj_ClientSrv Connection State.vi"("machine{connect}/VI{get state} name (local/no path resolution)"="DataLog Set Tag Value_srv.vi", "error in (no error)"=w924) -> ("server app ref"=w897:refnum<vi>, "resolved server path"=w896:path, "error out"=w895:errorcluster)  [unwired: 6 in, 5 out]
        n425 = local read "set tag value"() -> (w899:T2)
        n426 = stacked-sequence {
          tunnel: [w964] -> w898
          tunnel: [w963] -> w900
          tunnel: w895 -> [w962]
          tunnel: w897 -> [w961]
          tunnel: w896 -> [w960]
          tunnel: w899 -> [w959]
          frame #0 {
            # "avoid LV8 complaints"
            n427 = Path to Array of Strings(0:w960) -> (2:w965:string[])  [unwired: 1 out]
            n428 = Array Size(array=w965) -> (size(s)=w966:i32)
            n429 = case shown="1" w966 {
              tunnel: w960 -> [w973 w979]
              tunnel: w961 -> [w971 w978]
              tunnel: [w969 w974] -> w964
              tunnel: [w967 w977] -> w963
              tunnel: w959 -> [w968 w976]
              tunnel: w962 -> [w970 w975]
              frame 1 {
                n430 = Path To String(path=w973) -> (string=w972:string)
                n431 = Open VI Reference(type specifier VI Refnum (for type only)=w968, application reference (local)=w971, vi path=w972, error in (no error)=w970) -> (vi reference=w969:T2, error out=w967:errorcluster)  [unwired: 2 in]
              }
              frame Default {
                n432 = Open VI Reference(type specifier VI Refnum (for type only)=w976, application reference (local)=w978, vi path=w979, error in (no error)=w975) -> (vi reference=w974:T2, error out=w977:errorcluster)  [unwired: 2 in]
              }
            }
          }
        }
        "set tag value" <- w898
        n433 = local read "tag subset last"() -> (w912:T5)
        n434 = call "Library Open VI Ref Error Clarifier.vi"("VI path"=w896, "called VI error (no error)"=w900) -> ("error out"=w921:errorcluster)  [unwired: 13 in]
        n435 = call "obj_ClientSrv Connection State.vi"("machine{connect}/VI{get state} name (local/no path resolution)"="DataLog Dump Tag Buffer_srv.vi", "error in (no error)"=w921) -> ("server app ref"=w890:refnum<vi>, "resolved server path"=w889:path, "error out"=w894:errorcluster)  [unwired: 6 in, 5 out]
        n436 = local read "dump tag buffer"() -> (w891:T1)
        n437 = stacked-sequence {
          tunnel: [w943] -> w892
          tunnel: [w942] -> w893
          tunnel: w894 -> [w941]
          tunnel: w890 -> [w940]
          tunnel: w889 -> [w939]
          tunnel: w891 -> [w938]
          frame #0 {
            # "avoid LV8 complaints"
            n438 = Path to Array of Strings(0:w939) -> (2:w944:string[])  [unwired: 1 out]
            n439 = Array Size(array=w944) -> (size(s)=w945:i32)
            n440 = case shown="1" w945 {
              tunnel: w939 -> [w952 w958]
              tunnel: w940 -> [w950 w957]
              tunnel: [w948 w953] -> w943
              tunnel: [w946 w956] -> w942
              tunnel: w938 -> [w947 w955]
              tunnel: w941 -> [w949 w954]
              frame 1 {
                n441 = Path To String(path=w952) -> (string=w951:string)
                n442 = Open VI Reference(type specifier VI Refnum (for type only)=w947, application reference (local)=w950, vi path=w951, error in (no error)=w949) -> (vi reference=w948:T1, error out=w946:errorcluster)  [unwired: 2 in]
              }
              frame Default {
                n443 = Open VI Reference(type specifier VI Refnum (for type only)=w955, application reference (local)=w957, vi path=w958, error in (no error)=w954) -> (vi reference=w953:T1, error out=w956:errorcluster)  [unwired: 2 in]
              }
            }
          }
        }
        "dump tag buffer" <- w892
        n444 = call "Library Open VI Ref Error Clarifier.vi"("VI path"=w889, "called VI error (no error)"=w893) -> ("error out"=w922:errorcluster)  [unwired: 13 in]
        n445 = call "obj_ClientSrv Connection State.vi"("machine{connect}/VI{get state} name (local/no path resolution)"="DataLog Database Infos_srv.vi", "error in (no error)"=w922) -> ("server app ref"=w916:refnum<vi>, "resolved server path"=w915:path, "error out"=w914:errorcluster)  [unwired: 6 in, 5 out]
        n446 = stacked-sequence {
          tunnel: [w1027] -> w907
          tunnel: [w1026] -> w918
          tunnel: w914 -> [w1025]
          tunnel: w916 -> [w1024]
          tunnel: w915 -> [w1023]
          tunnel: w917 -> [w1022]
          frame #0 {
            # "avoid LV8 complaints"
            n447 = Path to Array of Strings(0:w1023) -> (2:w1028:string[])  [unwired: 1 out]
            n448 = Array Size(array=w1028) -> (size(s)=w1029:i32)
            n449 = case shown="1" w1029 {
              tunnel: w1023 -> [w1036 w1042]
              tunnel: w1024 -> [w1034 w1041]
              tunnel: [w1032 w1037] -> w1027
              tunnel: [w1030 w1040] -> w1026
              tunnel: w1022 -> [w1031 w1039]
              tunnel: w1025 -> [w1033 w1038]
              frame 1 {
                n450 = Path To String(path=w1036) -> (string=w1035:string)
                n451 = Open VI Reference(type specifier VI Refnum (for type only)=w1031, application reference (local)=w1034, vi path=w1035, error in (no error)=w1033) -> (vi reference=w1032:T6, error out=w1030:errorcluster)  [unwired: 2 in]
              }
              frame Default {
                n452 = Open VI Reference(type specifier VI Refnum (for type only)=w1039, application reference (local)=w1041, vi path=w1042, error in (no error)=w1038) -> (vi reference=w1037:T6, error out=w1040:errorcluster)  [unwired: 2 in]
              }
            }
          }
        }
        "database infos" <- w907
        n453 = call "Library Open VI Ref Error Clarifier.vi"("VI path"=w915, "called VI error (no error)"=w918) -> ("error out"=w930:errorcluster)  [unwired: 13 in]
        n454 = call "obj_ClientSrv Connection State.vi"("machine{connect}/VI{get state} name (local/no path resolution)"="DataLog Tag Subset Last_srv.vi", "error in (no error)"=w930) -> ("server app ref"=w910:refnum<vi>, "resolved server path"=w909:path, "error out"=w911:errorcluster)  [unwired: 6 in, 5 out]
        n455 = stacked-sequence {
          tunnel: [w1006] -> w908
          tunnel: [w1005] -> w913
          tunnel: w911 -> [w1004]
          tunnel: w910 -> [w1003]
          tunnel: w909 -> [w1002]
          tunnel: w912 -> [w1001]
          frame #0 {
            # "avoid LV8 complaints"
            n456 = Path to Array of Strings(0:w1002) -> (2:w1007:string[])  [unwired: 1 out]
            n457 = Array Size(array=w1007) -> (size(s)=w1008:i32)
            n458 = case shown="1" w1008 {
              tunnel: w1002 -> [w1015 w1021]
              tunnel: w1003 -> [w1013 w1020]
              tunnel: [w1011 w1016] -> w1006
              tunnel: [w1009 w1019] -> w1005
              tunnel: w1001 -> [w1010 w1018]
              tunnel: w1004 -> [w1012 w1017]
              frame 1 {
                n459 = Path To String(path=w1015) -> (string=w1014:string)
                n460 = Open VI Reference(type specifier VI Refnum (for type only)=w1010, application reference (local)=w1013, vi path=w1014, error in (no error)=w1012) -> (vi reference=w1011:T5, error out=w1009:errorcluster)  [unwired: 2 in]
              }
              frame Default {
                n461 = Open VI Reference(type specifier VI Refnum (for type only)=w1018, application reference (local)=w1020, vi path=w1021, error in (no error)=w1017) -> (vi reference=w1016:T5, error out=w1019:errorcluster)  [unwired: 2 in]
              }
            }
          }
        }
        "tag subset last" <- w908
        n462 = call "Library Open VI Ref Error Clarifier.vi"("VI path"=w909, "called VI error (no error)"=w913) -> ("error out"=w929:errorcluster)  [unwired: 13 in]
        n463 = call "Library Log Error to Window.vi"("error in (no error)"=w929) -> ("dup error"=w928:errorcluster)  [unwired: 13 in, 1 out]
        n464 = Select(t=w936, s=w928, f=w935) -> (s? t:f=w937:T8[])
      }
      frame "init databases" {
        w1053 = T8[] [enum."cleanup"] items=["empty queue", "poll list", "poll live", "resize", "set database", "get subsets", "winnow list", "filter list", "subset list", "show list", "create tag", "create meta tag", "clone tag", "rename tag", "configure tag", "chart tag", "set tag", "stat tag", "delete tag", "ablement", "initialize", "init refs", "init databases", "init persist", "cleanup", "stop"] ("Array Constant")
        n465 = call "obj_ClientSrv Client Access State.vi"() -> ("certificate"=w1054:string, "error out"=w1057:errorcluster)  [unwired: 14 in]
        n466 = local read "databases"() -> (w1056:T4)
        n467 = call-by-ref "?"(reference=w1056, error in=w1057, "certificate in"=w1054) -> (error out=w1058:errorcluster, "database names"=w1044:string[], 15:"error out"=w1055:errorcluster)  [unwired: 13 in, 1 out]
        n468 = call "Library Remote Call Error Merger.vi"("call by reference node error"=w1058, "called VI error (no error)"=w1055) -> ("error out"=w1051:errorcluster)  [unwired: 13 in]
        n469 = property on="database" class="Ring (strict)"(error in=w1051, "Value"=0 ("index"), "Strings []"=w1044) -> (error out=w1049:errorcluster)  [unwired: 1 in, 1 out]
        n470 = call "Library Log Error to Window.vi"("error in (no error)"=w1049) -> ("dup error"=w1048:errorcluster)  [unwired: 13 in, 1 out]
        n471 = Select(t=w1053, s=w1048, f=w1043) -> (s? t:f=w1052:T8[])
      }
      frame "init persist" {
        w1061 = T8[] [enum."resize", enum."set database", enum."poll list"] items=["empty queue", "poll list", "poll live", "resize", "set database", "get subsets", "winnow list", "filter list", "subset list", "show list", "create tag", "create meta tag", "clone tag", "rename tag", "configure tag", "chart tag", "set tag", "stat tag", "delete tag", "ablement", "initialize", "init refs", "init databases", "init persist", "cleanup", "stop"] ("Array Constant")
        n472 = call "Libary Persist Position and Controls.vi"("action"=enum16{"save", "load"}."load") -> ()  [unwired: 13 in, 2 out]
        n473 = Build Array (concatenate)(w1061, w1063) -> (w1062:T8[])
      }
      frame "cleanup" {
        w1092 = T8[] [enum."stop"] items=["empty queue", "poll list", "poll live", "resize", "set database", "get subsets", "winnow list", "filter list", "subset list", "show list", "create tag", "create meta tag", "clone tag", "rename tag", "configure tag", "chart tag", "set tag", "stat tag", "delete tag", "ablement", "initialize", "init refs", "init databases", "init persist", "cleanup", "stop"] ("Array Constant")
        n474 = local read "dump tag buffer"() -> (w1073:T1)
        n475 = local read "database infos"() -> (w1087:T6)
        n476 = local read "tag subset last"() -> (w1088:T5)
        n477 = local read "set tag value"() -> (w1072:T2)
        n478 = local read "databases"() -> (w1081:T4)
        n479 = Reshape Array(w1091, 0 ("dimension size")) -> (w1086:T15[])
        n480 = call "Libary Persist Position and Controls.vi"("action"=enum16{"save", "load"}."save") -> ()  [unwired: 13 in, 2 out]
        n481 = call "obj_Library Session.vi"("method"=t_Library_Session_Methods."delist") -> ()  [unwired: 11 in, 4 out]
        n482 = Close Reference(reference=w1073) -> ()  [unwired: 1 in, 1 out]
        n483 = Close Reference(reference=w1072) -> ()  [unwired: 1 in, 1 out]
        n484 = Close Reference(reference=w1081) -> ()  [unwired: 1 in, 1 out]
        n485 = Close Reference(reference=w1088) -> ()  [unwired: 1 in, 1 out]
        n486 = Close Reference(reference=w1087) -> ()  [unwired: 1 in, 1 out]
        n487 = Reshape Array(w1083, 0 ("dimension size")) -> (w1082:T15[])
        n488 = property on="tag list" class="MCListbox (strict)"("Item Names"=string[][] [], "Active Cell:Active Cell"=cluster{i32, i32} {-2, -2} ("Active Cell"), "Active Cell:Cell Background Color"=u32 15790320, "Active Cell:Active Cell"=cluster{i32, i32} {-1, -2} ("Active Cell"), "Active Cell:Cell Background Color"=u32 11776947, "Top Left Visible Cell"=cluster{"Row":u32, "Column":u32} {"Row"=0, "Column"=0}) -> ()  [unwired: 2 in, 2 out]
      }
      frame "stop" {
        n489 = invoke class="VI" method="FP.Close"() -> ()  [unwired: 3 in, 3 out]
      }
    }
  }
